vi "DAS_DEVEL.vi"() -> ()   [LabVIEW 2012]
uses:
  <vilib>/Utility/error.llb/DialogType.ctl
  SITK/Documents/SIToolkit/LabVIEW/Examples2012_4_1_0_4/Open-Close/CamHandle.vi
panel:
  out "Elapsed Time":u32
  in  "error in (no error) 4":errorcluster
  in  "bUseBuffer0 5":bool
  in  "bUseBuffer1 5":bool
  in  "Record 5":bool
  in  "Image Saving":u16(ring)=1 items=["Don't Save", "Save CoolSnap", "Save Pixelfly"]
  out "Slave OK?":bool
  in  "error in (no error) 3":errorcluster
  in  "bUseBuffer0 4":bool
  in  "bUseBuffer1 4":bool
  in  "Record 4":bool
  out "Entries in DB String":i32
  out "Database OK?":bool
  in  "?":bool
  in  "?":u16(ring) items=["Initialization", "Bulb Trigger (3x)", "Free Run (Both Cameras)", "Bulb Trigger (1x)"]
  in  "Image Tabs":T1(tab)
  in  "Display Image":dbl(ring) items=["2014-12-05_14;15;13"]
  out "Normalized Image":dbl[][](graph)
  out "Atoms":i16[][](graph)
  out "No Atoms":i16[][](graph)
  out "Dark Field":i16[][](graph)
  out "CoolSnap Free Run":i32[][](graph)
  out "CoolSnap Single Shot":i32[][](graph)
  in  "Image Tabs 2":T1(tab)
  out "Intensity Graph":dbl[][](graph)
  out "PF Atoms":u16[][](graph)
  out "PF No Atoms":u16[][](graph)
  out "PF Dark":u16[][](graph)
  out "PixelFly Free Run":u16[][](graph)
  out "PixelFly Single Shot":u16[][](graph)
  in  "Record 3":bool
  in  "bUseBuffer1 3":bool
  in  "bUseBuffer0 3":bool
  in  "Record 2":bool
  in  "bUseBuffer1 2":bool
  in  "bUseBuffer0 2":bool
  in  "bUseBuffer0":bool
  in  "bUseBuffer1":bool
  in  "Open StructureIn":T2={"Size"=88, "InterfaceType"=0, "Camera Number"=0, "CameraNumAtInterface"=0, "OpenFlags"=[], "OpenDWFlags"=[], "OpenPtrs"=[]}
  out "Bits/pixel":u16
  out "BufNr1":i16
  out "BufNr0":i16
  in  "error in (no error)":errorcluster
  in  "Camera Handle 2":u32
  in  "File and Display Name 2":string
  in  "error in (no error) 2":errorcluster
  in  "Errors":errorcluster
  in  "?":T3(tab)
  in  "Scaling":dbl(slide)=0.0016108638057548662 scale=0.001..0.1
  in  "PF Scale":dbl(slide)=0.9838778342396336 scale=0.001..10.0
  out "Database Output":string
  in  "ADC Gain":i32=-1 min=-1 step=1
  in  "ADC Speed":i32=-1 min=-3 step=1
  in  "Exposure (sec)":dbl format="%.3f"
  in  "Number of Images":u32=1
  in  "Number of Accumulations":u32=1
  in  "Acquire / Focus Flag":u32(ring)=2 items=["Synchronous Focus Mode"=1, "Synchronous NFrame Mode"=2, "Asynchronous Mode"=3, "Sequence Mode"=4]
  in  "Timing Mode":u32(ring)=4 items=["Free Run"=1, "Trigger First"=2, "Strobe"=3, "Bulb"=4, "Variable"=5, "Flash"=6]
  in  "Trigger Edge":u32(ring)=1 items=["Rising"=1, "Falling"=2]
  in  "Milliseconds Between Shots":u32=200
  in  "TriggerMode":u16(ring)=2 items=["Auto", "Software", "External sequence start ", "External exposure control"]
  in  "StorageMode":bool
  in  "Delay":u32=200
  in  "Exposure":u32=60
  in  "ExposureTimeBase":u16(ring)=1 items=["nanoseconds", "microseconds", "milliseconds"]
  in  "DelayTimeBase":u16(ring)=2 items=["nanoseconds", "microseconds", "milliseconds"]
  in  "ROIX0":u16=1 min=1
  in  "ROIY0":u16=1 min=1
  in  "ROIY1":u16=1 min=1
  in  "ROIX1":u16=1 min=1
  in  "Rate":i32
  in  "InterfaceType":u16(ring)=6 items=["IEEE1394 - Firewire", "IEEE1394/Firewire", "Matrox Helios Camera Link", "Silicon Software ME3 Camera Link", "National Instruments Camera Link", "Gigabit Ethernet", "USB", "Reserved", "Reserved", "Reserved", "Generic Camera Link with CLSER.DLL"]
  out "Top of Chamber Monitor":dynamicdata(graph)
  out "Bottom Cage Intensity Monitor":dynamicdata(graph)
  # "Stop Button"
  # "DAS Mode Select"
  # "Always run once in initialization mode before\nswitching modes. Be sure to change the camera\nsettings before running in a new mode."
  # "Images can only be saved when running \nin Bulb Trigger (3x) mode."
  # "CoolSnap HQ"
  # "CoolSnap HQ"
  # "CoolSnap HQ"
  # "CoolSnap HQ"
  # "CoolSnap HQ"
  # "CoolSnap HQ"
  # "PixelFly"
  # "PixelFly"
  # "PixelFly"
  # "PixelFly"
  # "PixelFly"
  # "PixelFly"
  # "Basic Setup"
  # "For Free Run:\n1) Synchronous Focus Mode\n2) Timing Mode: Free Run\n\nFor Bulb Trigger:\n1) Synchronous NFrame Mode\n2) Timing Mode: Bulb Trigger"
  # "Triggering Setup"
  # "Advanced Setup"
  # "For everyday use, Number of Accumulations should be 1"
  # "Basic Setup for PixelFly"
  # "For Free Run:\n1) Trigger Mode: Auto\n\nFor Bulb Trigger:\n1) Trigger Mode: External Sequence Start"
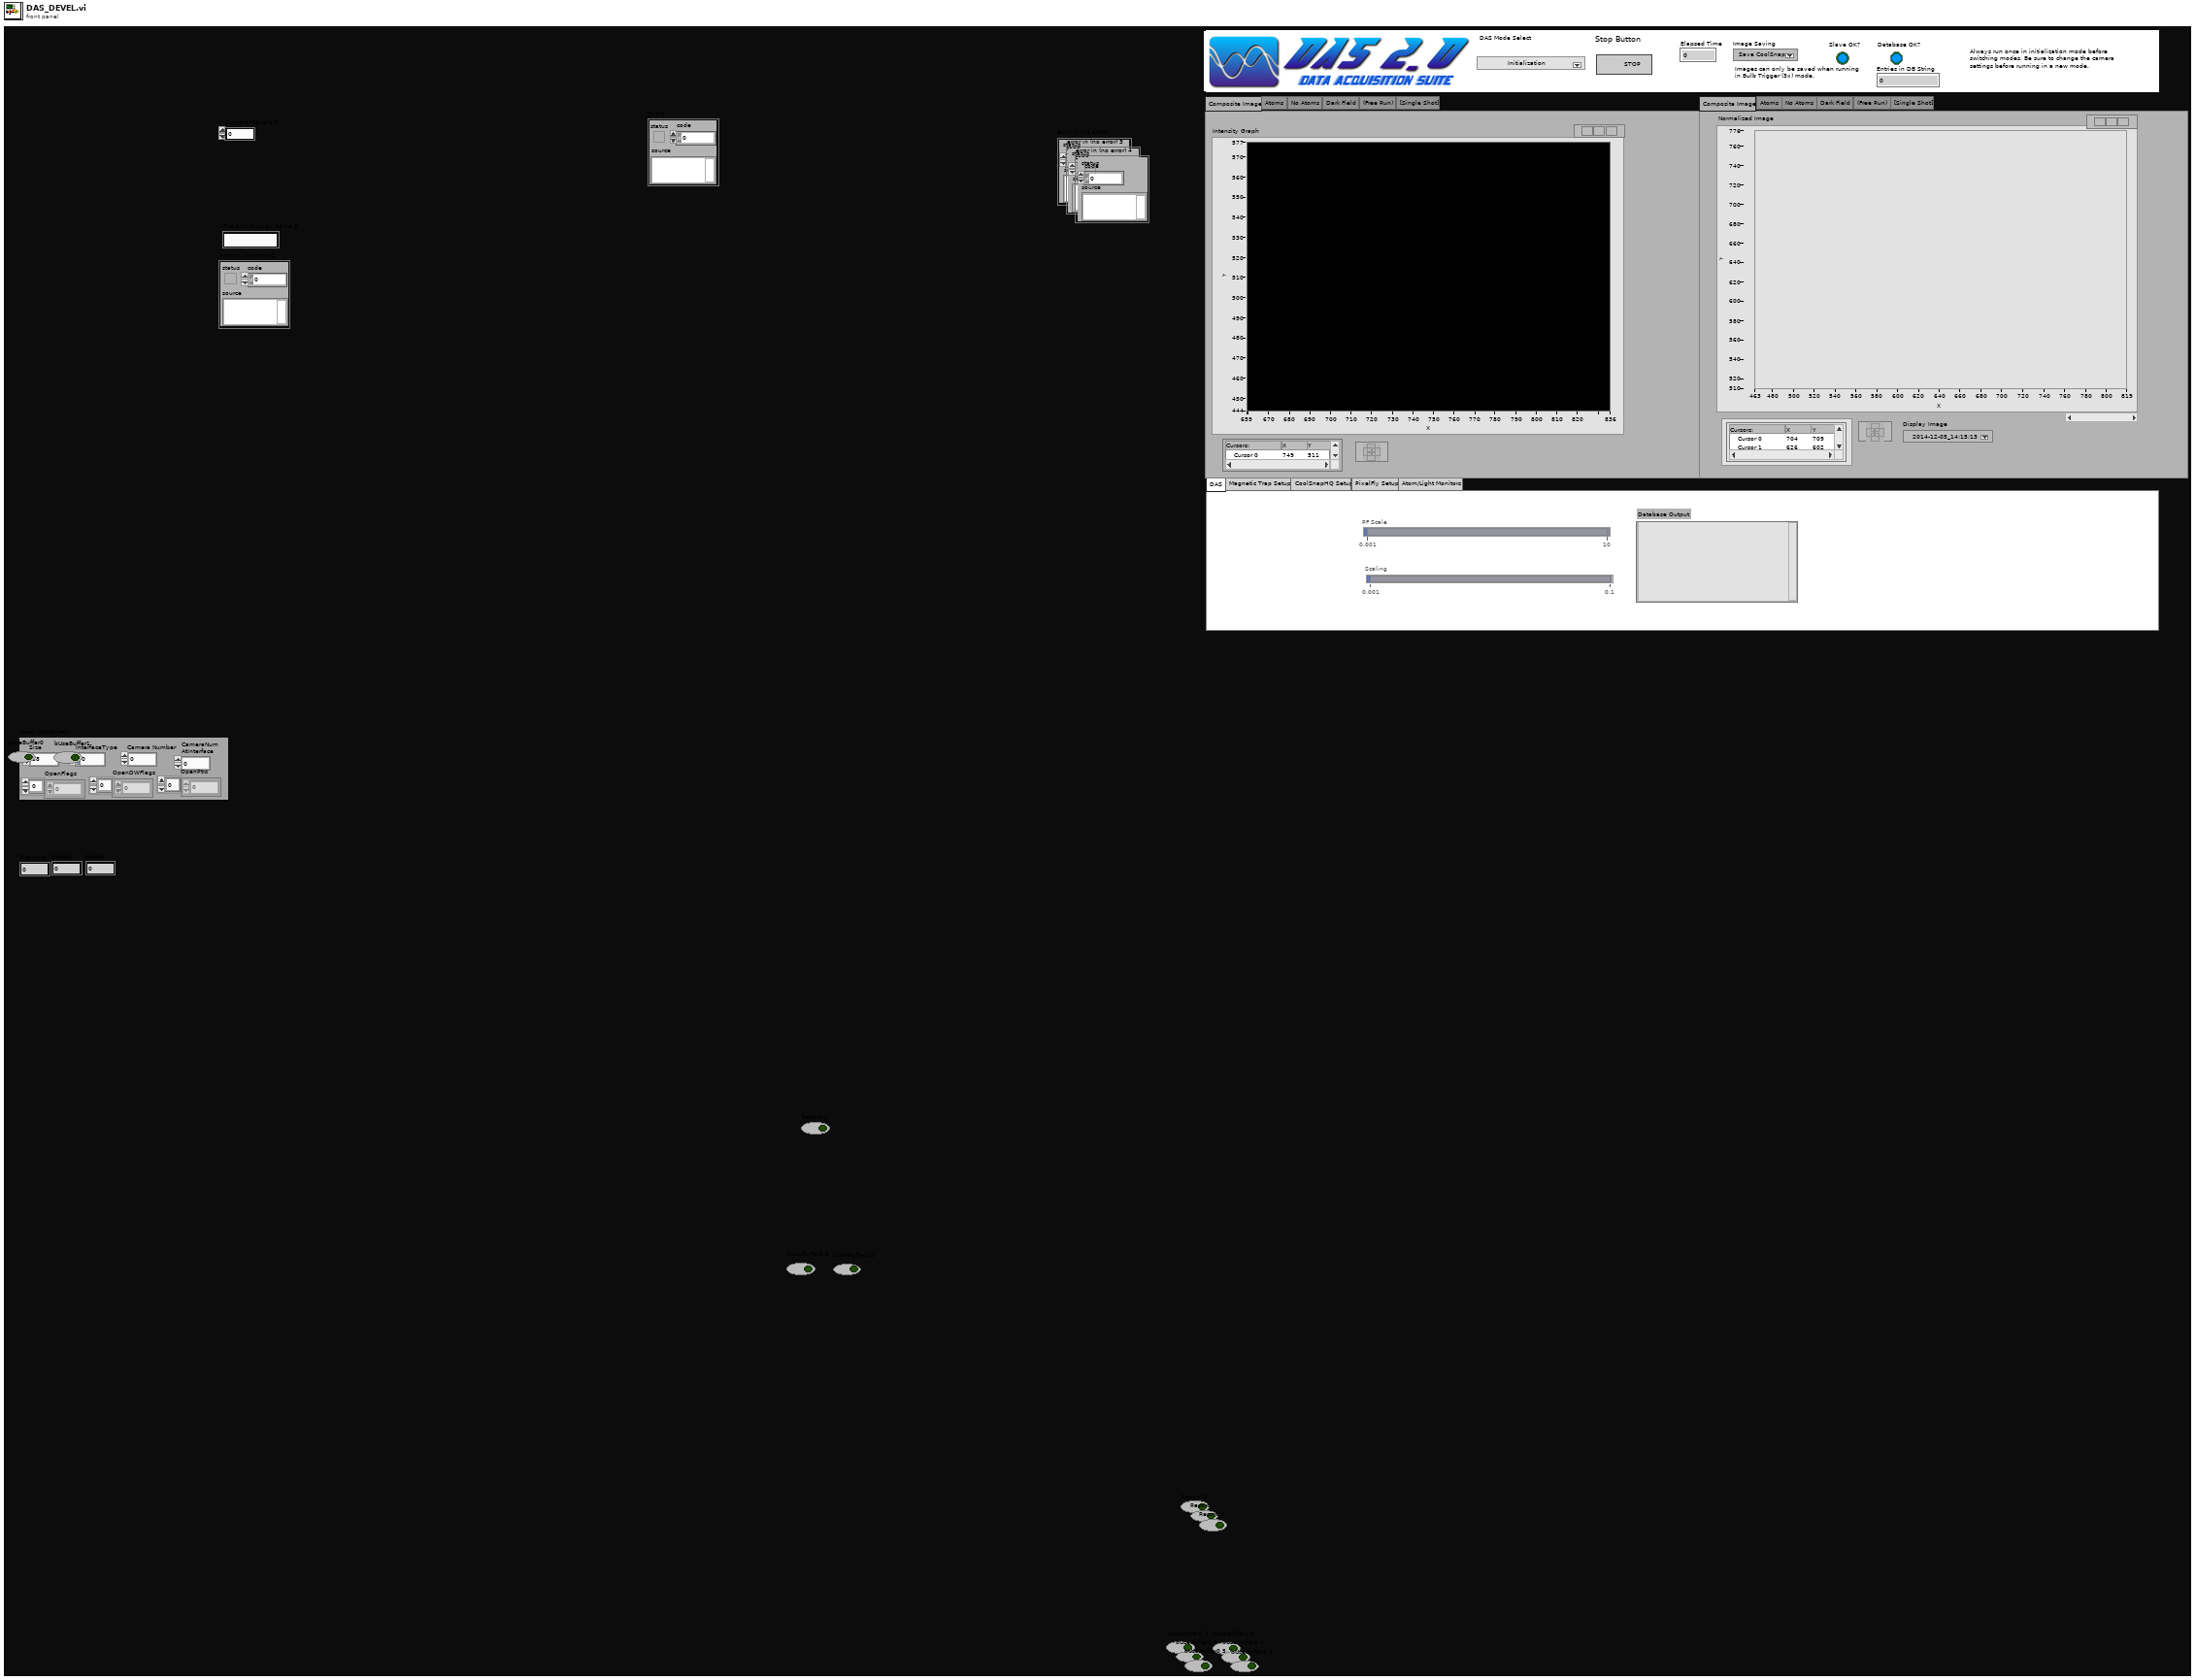
[diagram p1: front panel]
types:
  T1 = enum32{"Composite Image", "Atoms", "No Atoms", "Dark Field", "(Free Run)", "[Single Shot]"}
  T2 = cluster{"Size":u16, "InterfaceType":u16, "Camera Number":u16, "CameraNumAtInterface":u16, "OpenFlags":u16[], "OpenDWFlags":u32[], "OpenPtrs":u32[]}
  T3 = enum32{"DAS", "Magnetic Trap Setup", "CoolSnapHQ Setup", "PixelFly Setup", "Atom/Light Monitors"}
  T4 = enum16{"open", "replace", "create", "open or create", "replace or create", "replace or create with confirmation"}
  T5 = enum16{"big-endian, network order", "native, host order", "little-endian"}
  T6 = typedef "DialogType.ctl" = u16
  T7 = cluster{"Size":u16, "CamType":u16, "CamSubType":u16, "SerialNumber":u32, "HWVersion":u32, "FWVersion":u32, "InterfaceType":u16, "HardwareVersion":cluster{"BoardNum":u16, "HWVersions":cluster{"BoardName":string, "BatchNumber":u16, "MinorRevision":u8, "MajorRevision":u8, "Variant":u16}[]}, "FirmwareVersion":cluster{"DeviceNum":u16, "FWVersions":cluster{"DeviceName":string, "MinorRevision":u8, "MajorRevision":u8, "Variant":u16}[]}}
  T8 = cluster{"Size":u16, "SensorTypeDESC":u16, "SensorSubtypeDESC":u16, "MaxHorizontalResStdDESC":u16, "MaxVerticalResStdDESC":u16, "MaxHorizontalResExtDESC":u16, "MaxVerticalResExtDESC":u16, "DynResDESC":u16, "MaxBinHorzDESC":u16, "BinHorzStepDESC":bool, "MaxBinVertDESC":u16, "BinVertStepDESC":bool, "ROIHorzStepDESC":u16, "ROIVertStepDESC":u16, "NumADCDESC":u16, "IRDESC":bool, "MinDelayDESC":u32, "MaxDelayDESC":u32, "MinDelayStepDESC":u32, "MinExpoDESC":u32, "MaxExpoDESC":u32, "MinExpoStepDESC":u32, "MinDelayIRDESC":u32, "MaxDelayIRDESC":u32, "MinExpoIRDESC":u32, "MaxExpoIRDESC":u32, "TimeTableDESC":bool, "DoubleImageDESC":bool, "MinCoolSetDESC":i16, "MaxCoolSetDESC":i16, "MDefaultCoolSetDESC":i16, "PowerDownModeDESC":bool, "OffsetRegDESC":bool, "ColorPattern":cluster{"UpperLeftColor":u8, "UpperRightColor":u8, "LowerLeftColor":u8, "LowerRightColor":u8}, "PatternTypeDESC":bool, "PixelRates":u32[], "CoversionFactors":u16[], "Reserved":u32[], "NoiseFilterCapable":bool, "HotPixelCapable":bool, "HotPixelWithNoiseFilter":bool, "ASCIITimeCapable":bool, "Extended Description":bool, "Get Extended":bool, "Reserved Flag 1":bool, "Reserved Flag 2":bool}
  T9 = cluster{"Camera Handle":u32, "File Handle":u32, "Display Handle":u32, "Image Handle":u32}
  T10 = cluster{u16[][], "XResAct":u16, "YResAct":u16, "BufNrOut":i16, "BufNrOut":i16, "ErrorOut":errorcluster, "hout":u64, "Bits/pixel":u16}
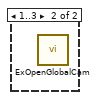
[diagram p3: hidden frame]
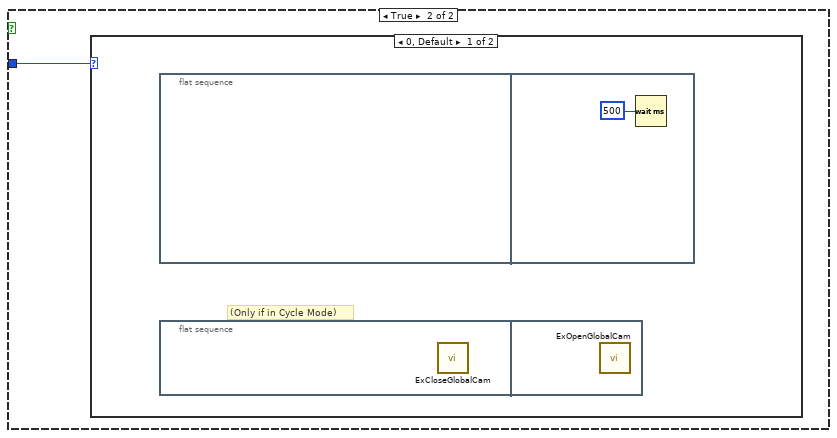
[diagram p4: hidden frame]
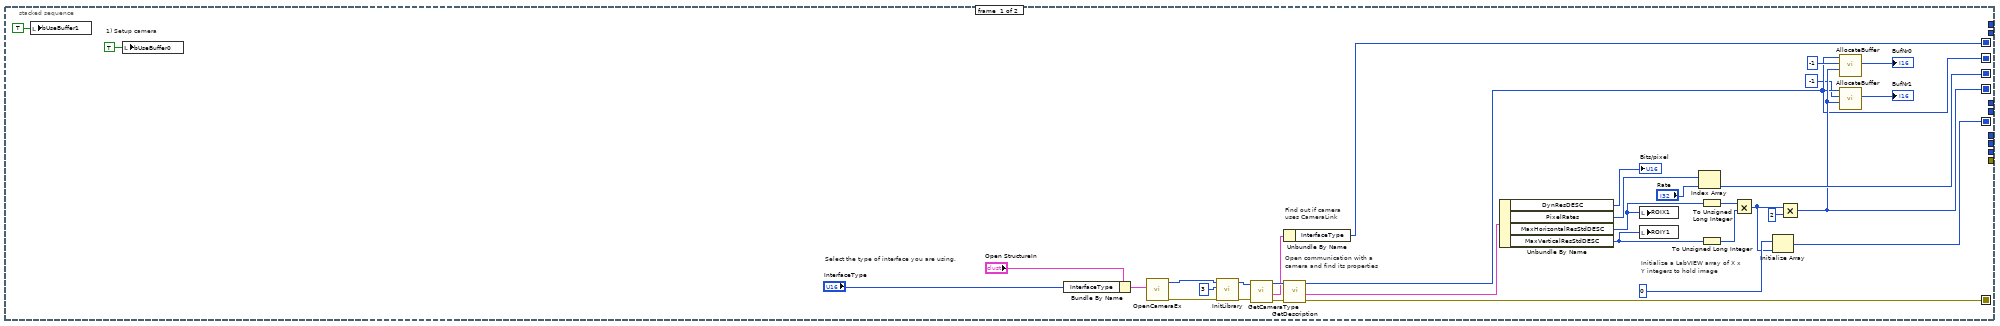
[diagram p6: hidden frame]
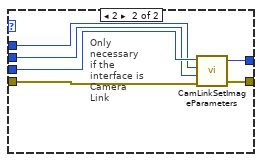
[diagram p7: hidden frame]
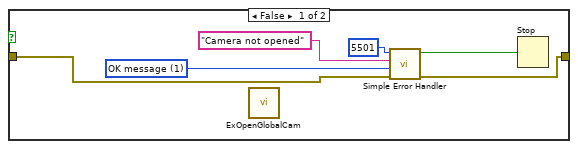
[diagram p9: hidden frame]
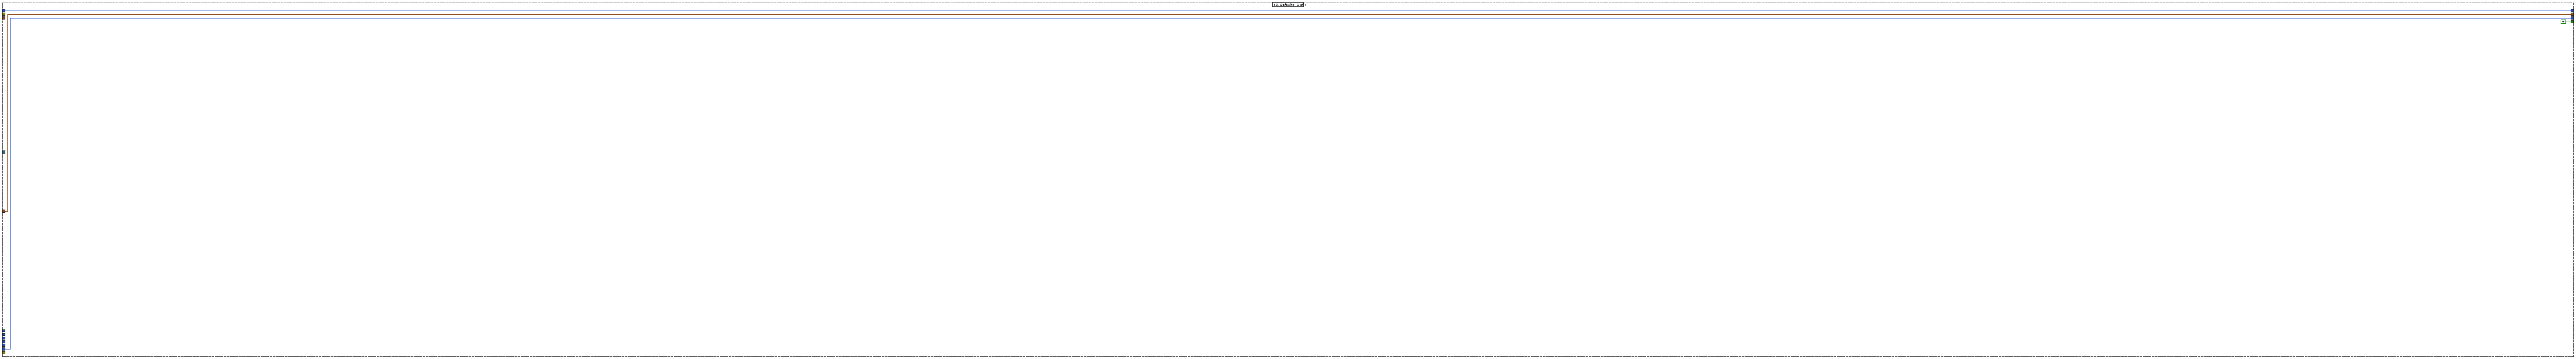
[diagram p10: hidden frame]
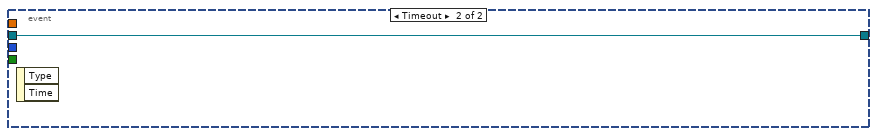
[diagram p13: hidden frame]
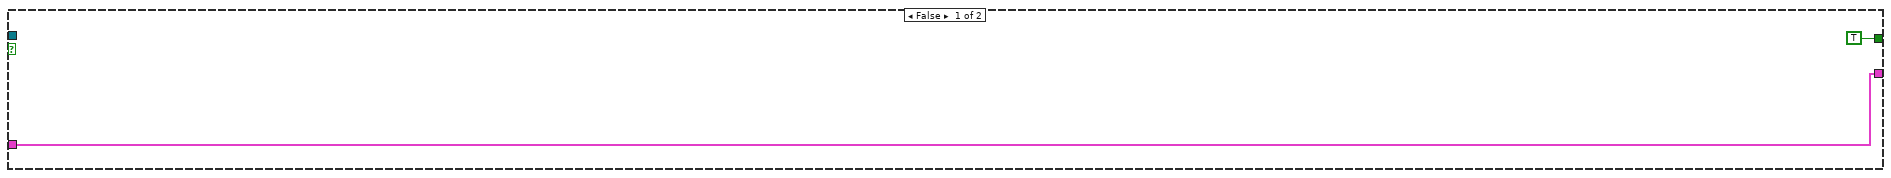
[diagram p14: hidden frame]
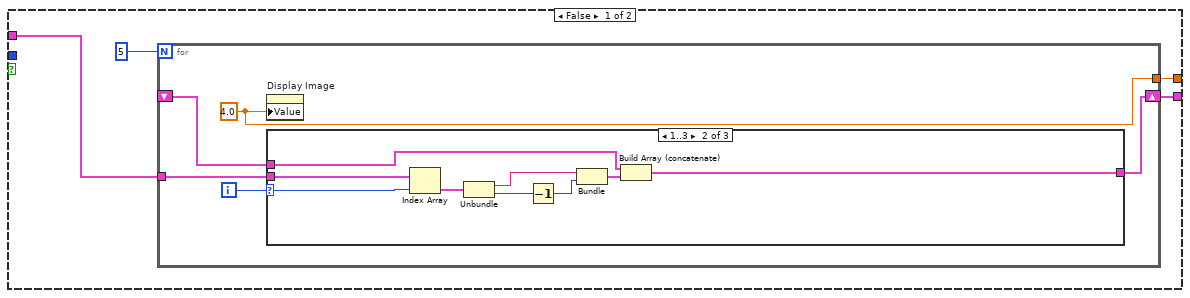
[diagram p16: hidden frame]
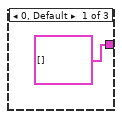
[diagram p17: hidden frame]
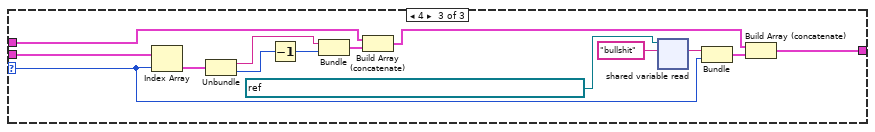
[diagram p18: hidden frame]
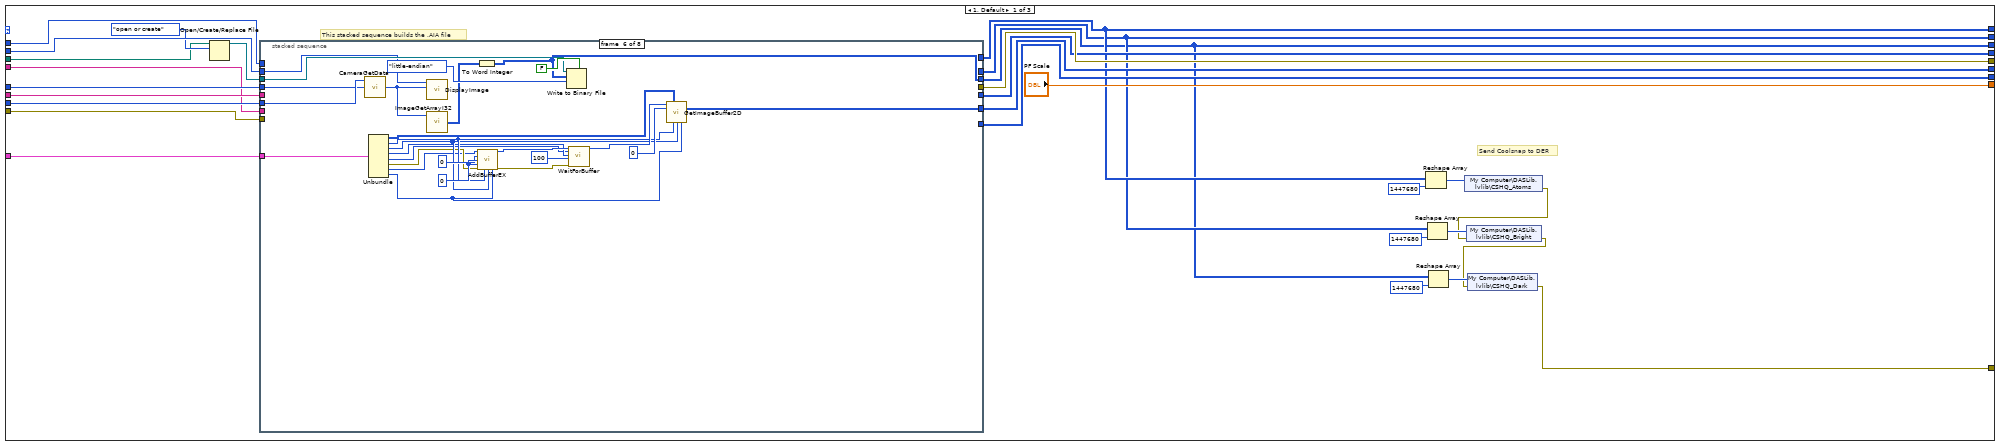
[diagram p20: hidden frame]
diagram:
  # "Tabs (Don't Touch These)"
  n1 = stacked-sequence {
    tunnel: [TRUE _] -> _
    tunnel: "?" -> [w3 _]
    tunnel: "?" -> [_ w51]
    frame #0 {
      # "Also, close any open displays to clean up the screen."
      # "Step 1:\nOpen the camera's global handle, if it is not already open."
      n2 = for {
        N: 10 -> [_]
        i -> [w8]
        w6 = T6 0 items=["no dialog", "OK message", "continue or stop message", "OK message + warnings", "continue/stop + warnings"] ("type of dialog (OK msg:1)")
        n3 = call <userlib>:"DisplayClose.vi"("Display Handle"=w8) -> ("error out"=w7:errorcluster)  [unwired: 1 in]
        n4 = call <vilib>:"General Error Handler.vi"("type of dialog (OK msg:1)"=w6, "error in (no error)"=w7) -> ()  [unwired: 9 in, 5 out]
      }
      n5 = global read "CamHandle.vi" "Camera Opened"() -> (w2:bool)
      n6 = case shown="False" w2 {
        tunnel: w3 -> [w9 w11]
        frame False {
          n7 = case shown="0, Default" w9 {
            frame 0, Default {
              n8 = flat-sequence {
                frame #0 {
                }
                frame #1 {
                  n9 = call <vilib>:"System Exec.vi"("command line"="\"C:\\Program Files\\Photometrics\\PVCam32\\utilities\\RSConfig\\RSConfig.exe\"") -> ()  [unwired: 7 in, 4 out]
                }
                frame #2 {
                  n10 = call "ExOpenGlobalCam.vi"() -> ()  [unwired: 1 in]
                }
              }
            }
            frame 1..3 {
              n11 = call "ExOpenGlobalCam.vi"() -> ()  [unwired: 1 in]
            }
          }
        }
        frame True {
          n12 = case shown="0, Default" w11 {
            frame 0, Default {
              # "(Only if in Cycle Mode)"
              n13 = flat-sequence {
                frame #0 {
                }
                frame #1 {
                  n14 = Wait (ms)(milliseconds to wait=u32 500) -> ()  [unwired: 1 out]
                }
              }
              n15 = flat-sequence {
                frame #0 {
                  n16 = call "ExCloseGlobalCam.vi"() -> ()  [unwired: 1 in]
                }
                frame #1 {
                  n17 = call "ExOpenGlobalCam.vi"() -> ()  [unwired: 1 in]
                }
              }
            }
            frame 1..3 {
            }
          }
        }
      }
    }
    frame #1 {
      w26 = u32 1  # Number Of Frames
      w27 = u32 4  # Display Type
      w28 = u32 2  # Data Type
      w30 = 13  # File Operations
      w31 = 67371008  # File Type
      w66 = u16 0 items=["Stop", "Run"] ("RecordingState")
      # "Create the Vision and Motion toolkit image(s)"
      # "Init the queue flags to FALSE"
      # "Initialize the CoolSnap Queues"
      # "Init for CoolSnap"
      # "Error Checking Sequence for CoolSnap\nCamera:"
      # "Initialization Sequence \nFor CoolSnap Camera:"
      # "This file not used"
      # "\"Build\" image and display handles"
      # "Set up display"
      # "Set up display"
      # "Step 2:\nSet up the experiment and take the images."
      # "For best performance."
      # "Execution:\n1) Outer case structure depends on DAS's state. When 0 (initialization), there is no DAQ loop.\n2) Main while loop is where DAQ and camera polling occur.\n3) Inner case structure responds to available images on camera. Hard-coded to build 3-image composite .AIA files.\n4) Innermost stacked sequence builds this .AIA file."
      # "CoolSnapHQ"
      # "Stop recording"
      n18 = flat-sequence {
        tunnel: ["Number of Images"] -> w59
        tunnel: [w183] -> w58
        tunnel: [w182] -> w57
        tunnel: [w197] -> w55
        tunnel: [w201] -> _
        tunnel: w59 -> [w201]
        tunnel: w58 -> [w200]
        tunnel: w57 -> [w199]
        tunnel: [w198] -> w54
        frame #0 {
        }
        frame #1 {
          n19 = global read "CamHandle.vi" "Cam Handle"() -> (w177:u32)
          n20 = call <userlib>:"CameraStop.vi"("Camera Handle"=w177) -> ("Camera Handle"=w178:u32)  [unwired: 1 in, 1 out]
          n21 = call <userlib>:"CameraADCset.vi"("ADC Gain"="ADC Gain", "ADC Speed"="ADC Speed", "Camera Handle"=w178) -> ("error out"=w194:errorcluster, "Camera Handle"=w196:u32)  [unwired: 3 in]
          n22 = call <userlib>:"CameraExperiment.vi"("Number of Accumulations"="Number of Accumulations", "Acquire / Focus Flag"="Acquire / Focus Flag", "error in"=w194, "Number of Images"="Number of Images", "Exposure (sec)"="Exposure (sec)", "Camera Handle"=w196) -> ("error out"=w188:errorcluster, "Camera Handle"=w189:u32)
          n23 = call <userlib>:"CameraTrigger.vi"("error in"=w188, "Trigger Edge"="Trigger Edge", "Timing Mode"="Timing Mode", "Camera Handle"=w189) -> ("error out"=w179:errorcluster, "Camera Handle"=w184:u32)
          n24 = call <userlib>:"CameraInitialize.vi"("error in"=w179, "Camera Handle"=w184) -> ("error out"=w181:errorcluster, "Camera Handle"=w180:u32)
          n25 = call <userlib>:"CameraStart.vi"("error in"=w181, "Camera Handle"=w180) -> ("error out"=w182:errorcluster, "Camera Handle"=w183:u32)
        }
        frame #2 {
          n26 = call <userlib>:"CameraCheckData.vi"("Camera Handle"=w200, "error in"=w199) -> ("Camera Handle"=w197:u32, "error out"=w198:errorcluster)  [unwired: 1 out]
        }
      }
      n27 = stacked-sequence {
        seq-local: [w100 _] -> [_ w158]
        seq-local: [w81 _] -> [_ _]
        seq-local: [w93 _] -> [_ w160]
        seq-local: [w80 _] -> [_ w155]
        seq-local: [w92 _] -> [_ w161]
        seq-local: [w91 _] -> [_ w159]
        tunnel: [_ w154] -> w50
        tunnel: [_ w150] -> w49
        tunnel: [_ w153] -> w48
        tunnel: [_ w152] -> w47
        tunnel: [_ w151] -> w46
        tunnel: [_ w149] -> w45
        tunnel: [_ w148] -> w44
        tunnel: [_ w147] -> w43
        frame #0 {
          # "Select the type of interface you are using."
          # "1) Setup camera"
          # "Find out if camera uses CameraLink"
          # "Initialize a LabVIEW array of X x Y integers to hold image"
          # "Open communication with a camera and find its properties"
          n28 = local write "bUseBuffer1"(TRUE) -> ()
          n29 = local write "bUseBuffer0"(TRUE) -> ()
          n30 = Bundle By Name(cluster="Open StructureIn", "InterfaceType"="InterfaceType") -> (w88:T2)
          n31 = call "OpenCameraEx.vi"("OpenStructureIn"=w88) -> ("error out"=w72:errorcluster, "hout"=w73:u64)  [unwired: 3 in, 2 out]
          n32 = call "InitLibrary.vi"("error in (no error)"=w72, "InterfaceType"=u32 3, "ph"=w73) -> ("error out"=w70:errorcluster, "hout"=w71:u64)  [unwired: 7 in]
          n33 = call "GetCameraType.vi"("ph"=w71, "error in (no error)"=w70) -> ("hout"=w97:u64, "CameraType"=w95:T7, "error out"=w96:errorcluster)  [unwired: 1 in, 1 out]
          n34 = Unbundle By Name(w95) -> ("InterfaceType"=w91:u16)
          n35 = call "GetDescription.vi"("ErrorIn"=w96, "ph"=w97) -> ("ErrorOut"=w92:errorcluster, "Description"=w99:T8, "hout"=w80:u64)  [unwired: 2 in, 1 out]
          n36 = Unbundle By Name(w99) -> ("DynResDESC"=→"Bits/pixel":u16, "PixelRates"=w94:u32[], "MaxHorizontalResStdDESC"=w86:u16, "MaxVerticalResStdDESC"=w85:u16)
          n37 = local write "ROIX1"(w86) -> ()
          n38 = local write "ROIY1"(w85) -> ()
          n39 = Index Array(array=w94, index="Rate") -> (element=w93:u32)
          n40 = To Unsigned Long Integer(number=w86) -> (unsigned 32bit integer=w83:u32)
          n41 = To Unsigned Long Integer(number=w85) -> (unsigned 32bit integer=w82:u32)
          n42 = Multiply(x=w83, y=w82) -> (x*y=w101:u32)
          n43 = Initialize Array(u16 0 ("Element Data"), w101) -> (w100:u16[])
          n44 = Multiply(x=w101, y=u32 2) -> (x*y=w81:u32)
          n45 = call "AllocateBuffer.vi"("Size"=w81, "BufNr"=i16 -1, "ph"=w80) -> ("BufNrOut"=→"BufNr0":i16)  [unwired: 3 in, 5 out]
          n46 = call "AllocateBuffer.vi"("Size"=w81, "BufNr"=-1, "ph"=w80) -> ("BufNrOut"=→"BufNr1":i16)  [unwired: 3 in, 5 out]
        }
        frame #1 {
          w146 = u16 1 items=["Stop", "Run"] ("RecordingState")
          # "Init for Pixelfly"
          # "Record images"
          # "Start recording"
          # "Allocate a buffer to store image data. to allocate a new buffer use buffer number = -1"
          # "Find size after arming"
          # "ArmCamera upolads all settings to the camera and prepares for new images"
          # "Find out if camera is recording, and stop it if it is"
          # "If required, insert more functions for binning.  etc. here"
          # "X x Y x 2 = number of bytes to store 1 image"
          # "Use a buffer queue to view images while recording. This is also used as \"live\" mode"
          # "Display while recording:"
          n47 = call "SetPixelRate.vi"("error in (no error)"=w161, "PixelRate"=w160, "ph"=w155) -> ("error out"=w144:errorcluster, "hout"=w145:u64)  [unwired: 2 in, 1 out]
          n48 = call "SetStorageMode.vi"("error in (no error)"=w144, "StorageMode"="StorageMode", "ph"=w145) -> ("error out"=w136:errorcluster, "hout"=w137:u64)  [unwired: 2 in, 1 out]
          n49 = call "SetTrigger.vi"("error in (no error)"=w136, "TriggerMode"="TriggerMode", "ph"=w137) -> ("error out"=w129:errorcluster, "hout"=w130:u64)  [unwired: 2 in, 1 out]
          n50 = call "SetDelayExposureTime.vi"("ph"=w130, "Delay"="Delay", "Exposure"="Exposure", "error in (no error)"=w129, "DelayTimeBase"="DelayTimeBase", "ExposureTimeBase"="ExposureTimeBase") -> ("hout"=w118:u64, "error out"=w116:errorcluster)  [unwired: 7 in, 1 out]
          n51 = call "SetROI.vi"("ph"=w118, "ROIX0"="ROIX0", "ROIY0"="ROIY0", "ROIX1"="ROIX1", "ROIY1"="ROIY1", "error in (no error)"=w116) -> ("hout"=w117:u64, "error out"=w115:errorcluster)  [unwired: 12 in]
          n52 = call "GetRecordingState.vi"("ErrorIn"=w115, "ph"=w117) -> ("ErrorOut"=w140:errorcluster, "RecordingState"=w142:u16, "hout"=w141:u64)  [unwired: 2 in, 1 out]
          n53 = case shown="1" w142 {
            tunnel: w141 -> [w171 w175]
            tunnel: w140 -> [w170 w174]
            tunnel: [w171 w173] -> w139
            tunnel: [w170 w172] -> w138
            frame 0, Default {
            }
            frame 1 {
              w176 = u16 0 items=["Stop", "Run"] ("RecordingState")
              n54 = call "SetRecordingState.vi"("ErrorIn"=w174, "RecordingState"=w176, "ph"=w175) -> ("ErrorOut"=w172:errorcluster, "hout"=w173:u64)  [unwired: 2 in, 1 out]
            }
          }
          n55 = local write "bUseBuffer0"(TRUE) -> ()
          n56 = local write "bUseBuffer1"(TRUE) -> ()
          n57 = call "ArmCamera.vi"("error in (no error)"=w138, "ph"=w139) -> ("error out"=w134:errorcluster, "hout"=w135:u64)  [unwired: 1 in, 1 out]
          n58 = call "GetSizes.vi"("ph"=w135, "ErrorIn"=w134) -> ("hout"=w131:u64, "XResAct"=w150:u16, "YResAct"=w153:u16, "ErrorOut"=w133:errorcluster)  [unwired: 11 in, 3 out]
          n59 = To Unsigned Long Integer(number=w150) -> (unsigned 32bit integer=w119:u32)
          n60 = To Unsigned Long Integer(number=w153) -> (unsigned 32bit integer=w120:u32)
          n61 = Multiply(x=w119, y=w120) -> (x*y=w121:u32)
          n62 = Multiply(x=w121, y=u32 2) -> (x*y=w106:u32)
          n63 = local read "BufNr0"() -> (w156:i16)
          n64 = call "AllocateBuffer.vi"("error in (no error)"=w133, "Size"=w106, "BufNr"=w156, "ph"=w131) -> ("error out"=w110:errorcluster, "BufNrOut"=w152:i16, "hout"=w108:u64)  [unwired: 2 in, 3 out]
          n65 = local read "BufNr1"() -> (w157:i16)
          n66 = call "AllocateBuffer.vi"("error in (no error)"=w110, "Size"=w106, "BufNr"=w157, "ph"=w108) -> ("error out"=w109:errorcluster, "BufNrOut"=w151:i16, "hout"=w107:u64)  [unwired: 2 in, 3 out]
          n67 = case shown="0, Default" w159 {
            tunnel: w109 -> [w162 w169]
            tunnel: [w162 w168] -> w124
            tunnel: w107 -> [w163 w167]
            tunnel: [w163 w166] -> w123
            tunnel: w153 -> [_ w165]
            tunnel: w150 -> [_ w164]
            frame 0, Default {
            }
            frame 2 {
              # "Only necessary if the interface is Camera Link"
              n68 = call "CamLinkSetImageParameters.vi"("error in (no error)"=w169, "YRes"=w165, "XRes"=w164, "ph"=w167) -> ("error out"=w168:errorcluster, "hout"=w166:u64)  [unwired: 1 out]
            }
          }
          n69 = local read "Bits/pixel"() -> (w147:u16)
          n70 = Reshape Array(w158, w153, w150) -> (w154:u16[][])
          n71 = call "SetRecordingState.vi"("ErrorIn"=w124, "RecordingState"=w146, "ph"=w123) -> ("ErrorOut"=w148:errorcluster, "hout"=w149:u64)  [unwired: 2 in, 1 out]
        }
      }
      n72 = Wait (ms)(milliseconds to wait=u32 5) -> ()  [unwired: 1 out]
      n73 = global read "CamHandle.vi" "Camera Opened"() -> (w41:bool)
      n74 = call <userlib>:"CameraGetDataDim.vi"("Camera Handle"="Camera Handle 2", "error in"="error in (no error) 2") -> ("Camera Handle"=w34:u32, "Xdim"=w21:u32, "Ydim"=w20:u32, "error out"=w39:errorcluster)
      n75 = while {
        tunnel: w21 -> [w210]
        tunnel: w20 -> [w209]
        tunnel: [w204] -> w25
        tunnel: [w203] -> w24
        i -> [w208]
        stop <- w205 continue-if-true
        w211 = 800
        n76 = Increment(x=w208) -> (x+1=w202:i32)
        n77 = Quotient & Remainder(x=w210, y=w202) -> (floor(x/y)=w204:u32)  [unwired: 1 out]
        n78 = Quotient & Remainder(x=w209, y=w202) -> (floor(x/y)=w203:u32)  [unwired: 1 out]
        n79 = Greater?(x=w204, y=w211) -> (0:w207:bool)
        n80 = Greater?(x=w203, y=w211) -> (0:w206:bool)
        n81 = Or(x=w207, y=w206) -> (x .or. y?=w205:bool)
      }
      n82 = case shown="True" w41 {
        tunnel: [w216 w218] -> _
        tunnel: "Errors" -> [w212 w218]
        frame False {
          w217 = u16 1 items=["no dialog", "OK message", "continue or stop message"] ("type of dialog (OK msg:1)")
          n83 = call "ExOpenGlobalCam.vi"() -> ()  [unwired: 1 in]
          n84 = call <vilib>:"Simple Error Handler.vi"("error code (no error:0)"=5501, "error source (\" \")"="Camera not opened", "type of dialog (OK msg:1)"=w217, "error in (no error)"=w212) -> ("error?"=w214:bool, "error out"=w216:errorcluster)  [unwired: 1 in, 3 out]
          n85 = Stop(stop? (T)=w214) -> ()
        }
        frame True {
        }
      }
      n86 = Obtain Queue(max queue size (-1, unlimited)=5, name (unnamed)="CSHQ_1", element data type=dbl[][] [] ("Normalized Image")) -> (queue out=w42:refnum<queue>)  [unwired: 2 in, 2 out]
      n87 = shared-variable-write(refnum<k21> "ni.var.psp://my computer/Untitled Library 1/CSHQ_1_Changed" ("shared variable refnum in"), FALSE) -> ()  [unwired: 1 in, 2 out]
      n88 = To Unsigned Long Integer(number=w25) -> (unsigned 32bit integer=w23:u32)
      n89 = To Unsigned Long Integer(number=w24) -> (unsigned 32bit integer=w22:u32)
      n90 = call <userlib>:"ImageCreate.vi"("X dimension"=w21, "Y dimension"=w20, "Data Type"=w28, "error in"=w39, "Number Of Frames"=w26) -> ("Image Handle"=w32:u32, "error out"=w38:errorcluster)
      n91 = call <userlib>:"DisplayOpen.vi"("Display Title"="File and Display Name 2", "Image Handle"=w32, "error in"=w38, "Display Height"=w22, "Display Width"=w23, "Display Type"=w27) -> ("error out"=w37:errorcluster, "Display Handle"=w18:u32)
      n92 = call <userlib>:"FileOpen.vi"("error in"=w37, "File Operations"=w30, "FileName"="File and Display Name 2", "File Type"=w31) -> ("File Handle"=w33:u32)  [unwired: 1 out]
      n93 = Bundle("Camera Handle"=w34, "File Handle"=w33, "Display Handle"=w18, "Image Handle"=w32) -> (w53:T9)  [unwired: 1 in]
      n94 = Bundle("Xdim"=w21, "Ydim"=w20, 0) -> (w56:cluster{"Xdim":u32, "Ydim":u32, i32})  [unwired: 1 in]
      n95 = case shown="1" w51 {
        selector: w51 -> [_ w234 w1045 w1132]
        tunnel: w53 -> [w222 w236 w1047 w1134]
        tunnel: [w222 w236 w1047 w1134] -> w69
        tunnel: w55 -> [w221 w241 w1052 w1139]
        tunnel: w54 -> [_ _ _ _]
        tunnel: [w221 w241 w1052 w1139] -> _
        tunnel: [TRUE FALSE FALSE FALSE] -> _
        tunnel: w56 -> [_ _ _ _]
        tunnel: w50 -> [_ w233 w1044 w1131]
        tunnel: w49 -> [_ w232 w1043 w1130]
        tunnel: w48 -> [_ w231 w1042 w1129]
        tunnel: w47 -> [_ w230 w1041 w1128]
        tunnel: w46 -> [_ w229 w1040 w1127]
        tunnel: w45 -> [w219 w228 w1039 w1126]
        tunnel: w44 -> [_ w227 w1038 w1125]
        tunnel: w43 -> [_ w226 w1037 w1124]
        tunnel: [w219 w225 w1036 w1123] -> w65
        tunnel: w42 -> [_ w224 _ _]
        frame 0, Default {
        }
        frame 1 {
          n96 = Unbundle(w236) -> ("Camera Handle"=w235:u32, "File Handle"=w239:u32, "Display Handle"=w238:u32, "Image Handle"=w237:u32)
          n97 = while {
            tunnel: "error in (no error)" -> [w290]
            tunnel: w235 -> [w289]
            tunnel: [w286] -> _
            tunnel: w239 -> [_]
            tunnel: w238 -> [w285]
            tunnel: w237 -> [w284]
            tunnel: [w282] -> _
            tunnel: w234 -> [w276]
            tunnel: w233 -> [w272]
            tunnel: w232 -> [w271]
            tunnel: w231 -> [w270]
            tunnel: w230 -> [w268]
            tunnel: w229 -> [w269]
            tunnel: w228 -> [w264]
            tunnel: w227 -> [w267]
            tunnel: w226 -> [w266]
            tunnel: [w264] -> w225
            shift-right: [w263] -> _
            shift-left: w224 -> [w249]
            shift-right: [w256] -> _
            shift-left: cluster{"date/time string":string, i32}[] [] -> [w257]
            stop <- w275 continue-if-true
            (unwired) 1
            # "Destroy the buffer,\nfind the right image,\nrebuild the buffer"
            # "Cluster for PixelFly"
            # "PixelFly Camera Functions"
            # "NI Scope"
            # "CoolSnap Camera Functions"
            # "ADC Inputs"
            # "THIS is the main loop.\nPoll the camera continuously while other data is taken in."
            n98 = Bundle(w272, "XResAct"=w271, "YResAct"=w270, "BufNrOut"=w269, "BufNrOut"=w268, "ErrorOut"=w267, "hout"=w264, "Bits/pixel"=w266) -> (w265:T10)  [unwired: 1 in]
            n99 = call <userlib>:"CameraCheckData.vi"("Camera Handle"=w289, "error in"=w290) -> ("Camera Handle"=w288:u32, "Number Of Frames Available"=w281:i32, "error out"=w287:errorcluster)
            n100 = Wait Until Next ms Multiple(millisecond multiple=1) -> (millisecond timer value=w282:u32)
            "Elapsed Time" <- w282
            n101 = Not(x="?") -> (.not. x?=w274:bool)
            n102 = Greater Or Equal?(x=w281, y=1) -> (x >= y?=w279:bool)
            n103 = Greater?(x=w276, y=u16 0) -> (0:w247:bool)
            n104 = call "DAQ Assistant"() -> ("data"=w243:dynamicdata)  [unwired: 17 in, 2 out]
            n105 = And(x=w247, y=w274) -> (x .and. y?=w275:bool)
            n106 = Split Signals(w243) -> (w245:dynamicdata, →"Bottom Cage Intensity Monitor":dynamicdata)  [unwired: 2 in]
            n107 = case shown="True" w279 {
              selector: w279 -> [w387 _]
              tunnel: w288 -> [_ w456]
              tunnel: w287 -> [w388 w455]
              tunnel: [w387 TRUE] -> _
              tunnel: [w388 w448] -> w286
              tunnel: w285 -> [_ w454]
              tunnel: w284 -> [_ w451]
              tunnel: w282 -> [_ _]
              tunnel: w265 -> [_ w440]
              tunnel: w249 -> [w386 w418]
              tunnel: [w386 w416] -> w250
              tunnel: "Image Saving" -> [_ w411]
              frame False {
              }
              frame True {
                w422 = 0 ("y")
                # "Enter this loop when image data is available on the coolsnap"
                # "Add new image to \"top\" of queue"
                # "Save Images?"
                n108 = Get Queue Status(queue=w418) -> (queue out=w417:refnum<queue>, # elements in queue=w421:i32)  [unwired: 2 in, 6 out]
                n109 = Less?(x=w421, y=5) -> (x < y?=w419:bool)
                n110 = Get Date/Time In Seconds() -> (seconds since 1Jan1904=w442:timestamp)
                n111 = Format Date/Time String(time format string (%c)="%Y-%m-%d_%H;%M;%S", seconds (now)=w442) -> (date/time string=w413:string)  [unwired: 1 in]
                n112 = Concatenate Strings("Z:\\Current\\" ("string"), w413, ".aia" ("string")) -> (w449:string)
                n113 = String To Path(string=w449) -> (path=w410:path)
                n114 = call <vilib>:"System Exec.vi"("command line"="php C:\\Users\\BECV\\Documents\\GitHub\\DAS\\dbquery.php") -> ("standard output"=w399:string)  [unwired: 7 in, 3 out]
                n115 = case shown="2" w411 {
                  tunnel: w456 -> [w484 w669 w851]
                  tunnel: w455 -> [w483 w668 w850]
                  tunnel: w454 -> [w482 w667 w849]
                  tunnel: w451 -> [w481 w666 w848]
                  tunnel: w410 -> [w471 w657 _]
                  tunnel: [w480 w665 w841] -> w448
                  tunnel: "Milliseconds Between Shots" -> [w479 w664 w847]
                  tunnel: w440 -> [w478 w663 w846]
                  tunnel: [w459 w662 w830] -> w395
                  tunnel: [w458 w661 w829] -> w394
                  tunnel: [w457 w660 w827] -> w392
                  tunnel: [w477 w644 w845] -> w435
                  tunnel: [w476 w643 w844] -> w432
                  tunnel: [w475 w642 w828] -> w429
                  tunnel: ["PF Scale" w654 w840] -> w426
                  tunnel: w413 -> [w469 w655 w843]
                  tunnel: w399 -> [w473 w659 w842]
                  tunnel: [w460 w645 errorcluster {"status"=FALSE, "code"=0, "source"=""} ("error IO")] -> w391
                  frame 1, Default {
                    # "Send Coolsnap to DER"
                    # "This stacked sequence builds the .AIA file"
                    n116 = Open/Create/Replace File(file path (use dialog)=w471, operation (0:open)=T4."open or create") -> (refnum out=w470:refnum<file>)  [unwired: 4 in, 2 out]
                    n117 = stacked-sequence {
                      tunnel: w484 -> [_ w538 _ w571 _ w601 _ _]
                      tunnel: w483 -> [_ _ _ _ _ _ _ _]
                      tunnel: w482 -> [_ w540 _ w568 _ w598 _ _]
                      tunnel: w481 -> [_ w539 _ w567 _ w597 _ _]
                      tunnel: w470 -> [w498 w532 _ w569 _ w599 w610 w641]
                      tunnel: [_ w535 _ _ _ _ _ _] -> w480
                      tunnel: w479 -> [_ _ w542 _ w572 _ _ _]
                      tunnel: [_ w516 _ _ _ _ _ _] -> w459
                      tunnel: [_ _ _ w563 _ _ _ _] -> w458
                      tunnel: [_ _ _ _ _ w593 _ _] -> w457
                      tunnel: w478 -> [_ w500 _ w547 _ w577 _ _]
                      tunnel: [_ w499 _ _ _ _ _ _] -> w477
                      tunnel: [_ _ _ w546 _ _ _ _] -> w476
                      tunnel: [_ _ _ _ _ w576 _ _] -> w475
                      tunnel: w469 -> [_ _ _ _ _ _ w608 _]
                      tunnel: w473 -> [_ _ _ _ _ _ w604 _]
                      frame #0 {
                        # "AIA, 16 bit, NULL"
                        n118 = Write to Binary File(file (use dialog)=w498, data="AIA", 5:FALSE ("prepend array or string size? (T)"), 9:T5."little-endian" ("byte order (0:big-endian, network order)")) -> (refnum out=w494:refnum<file>)  [unwired: 2 in, 2 out]
                        n119 = To Byte Integer(number=2) -> (8bit integer=w487:i8)
                        n120 = Write to Binary File(file (use dialog)=w494, data=w487, 5:FALSE ("prepend array or string size? (T)"), 9:T5."little-endian" ("byte order (0:big-endian, network order)")) -> (refnum out=w493:refnum<file>)  [unwired: 2 in, 2 out]
                        n121 = To Byte Integer(number=0) -> (8bit integer=w485:i8)
                        n122 = Write to Binary File(file (use dialog)=w493, data=w485, 5:FALSE ("prepend array or string size? (T)"), 9:T5."little-endian" ("byte order (0:big-endian, network order)")) -> ()  [unwired: 2 in, 3 out]
                      }
                      frame #1 {
                        w511 = 0
                        w525 = T5."little-endian" ("byte order (0:big-endian, network order)")
                        n123 = call <userlib>:"CameraGetData.vi"("Data Handle"=w539, "Camera Handle"=w538) -> ("error out"=w541:errorcluster, "Data Handle"=w536:u32)  [unwired: 1 in, 1 out]
                        n124 = Unbundle(w500) -> (w508:u16[][], "XResAct"=w507:u16, "YResAct"=w506:u16, "BufNrOut"=w505:i16, "BufNrOut"=w504:i16, "ErrorOut"=w503:errorcluster, "hout"=w502:u64, "Bits/pixel"=w501:u16)
                        n125 = call <userlib>:"DisplayImage.vi"("error in"=w541, "Image Handle"=w536, "Display Handle"=w540) -> ()  [unwired: 1 in, 2 out]
                        n126 = call <userlib>:"ImageGetArrayI32.vi"("Image Handle"=w536) -> ("Array int 32"=w517:i32[][])  [unwired: 2 in, 2 out]
                        n127 = To Word Integer(number=w517) -> (16bit integer=w516:i16[][])
                        n128 = Array Size(array=w517) -> (size(s)=w518:i32[])
                        n129 = call "AddBufferEX.vi"("ph"=w502, "BuffNr"=i16 0, "1stImage"=w511, "LastImage"=w511, "error in (no error)"=w503, "XRes"=w507, "YRes"=w506, "BitPerPixel"=w501) -> ("hout"=w513:u64, "error out"=w512:errorcluster)  [unwired: 5 in, 1 out]
                        n130 = Index Array(array=w518, index=0) -> (element=w523:i32)
                        n131 = Index Array(array=w518, index=1) -> (element=w522:i32)
                        n132 = call "WaitForBuffer.vi"("ph"=w513, "sBufNr"=w504, "sBufNr 2"=w505, "timeout"=100, "error in (no error)"=w512) -> ("hout"=w515:u64)  [unwired: 10 in, 4 out]
                        n133 = To Word Integer(number=w523) -> (16bit integer=w524:i16)
                        n134 = To Word Integer(number=w522) -> (16bit integer=w521:i16)
                        n135 = Write to Binary File(file (use dialog)=w532, data=w524, 5:FALSE ("prepend array or string size? (T)"), 9:w525) -> (refnum out=w531:refnum<file>)  [unwired: 2 in, 2 out]
                        n136 = call "GetImageBuffer2D.vi"("ph"=w515, "BuffIn"=w508, "BuffNr"=i16 0, "xRes"=w507, "yRes"=w506, "Bitresolution"=w501) -> ("BuffOut"=w499:u16[][])  [unwired: 6 in, 3 out]
                        n137 = Write to Binary File(file (use dialog)=w531, data=w521, 5:FALSE ("prepend array or string size? (T)"), 9:w525) -> (refnum out=w530:refnum<file>)  [unwired: 2 in, 2 out]
                        n138 = To Word Integer(number=3 ("index")) -> (16bit integer=w520:i16)
                        n139 = Write to Binary File(file (use dialog)=w530, data=w520, 5:FALSE ("prepend array or string size? (T)"), 9:w525) -> (refnum out=w529:refnum<file>)  [unwired: 2 in, 2 out]
                        n140 = Write to Binary File(file (use dialog)=w529, data=w516, 5:FALSE ("prepend array or string size? (T)"), 9:w525) -> (error out=w535:errorcluster)  [unwired: 2 in, 2 out]
                      }
                      frame #2 {
                        n141 = Quotient & Remainder(x=w542, y=u32 10) -> (floor(x/y)=w543:u32)  [unwired: 1 out]
                        n142 = Add(x=w543, y=w542) -> (x+y=w545:u32)
                        n143 = Wait (ms)(milliseconds to wait=w545) -> ()  [unwired: 1 out]
                      }
                      frame #3 {
                        w558 = 0
                        n144 = call <userlib>:"CameraGetData.vi"("Data Handle"=w567, "Camera Handle"=w571) -> ("Data Handle"=w566:u32)  [unwired: 1 in, 2 out]
                        n145 = Unbundle(w547) -> (w555:u16[][], "XResAct"=w554:u16, "YResAct"=w553:u16, "BufNrOut"=w552:i16, "BufNrOut"=w551:i16, "ErrorOut"=w550:errorcluster, "hout"=w549:u64, "Bits/pixel"=w548:u16)
                        n146 = call <userlib>:"DisplayImage.vi"("Image Handle"=w566, "Display Handle"=w568) -> ()  [unwired: 2 in, 2 out]
                        n147 = call <userlib>:"ImageGetArrayI32.vi"("Image Handle"=w566) -> ("Array int 32"=w564:i32[][])  [unwired: 2 in, 2 out]
                        n148 = To Word Integer(number=w564) -> (16bit integer=w563:i16[][])
                        n149 = call "AddBufferEX.vi"("ph"=w549, "BuffNr"=i16 0, "1stImage"=w558, "LastImage"=w558, "error in (no error)"=w550, "XRes"=w554, "YRes"=w553, "BitPerPixel"=w548) -> ("hout"=w560:u64, "error out"=w559:errorcluster)  [unwired: 5 in, 1 out]
                        n150 = Write to Binary File(file (use dialog)=w569, data=w563, 5:FALSE ("prepend array or string size? (T)"), 9:T5."little-endian" ("byte order (0:big-endian, network order)")) -> ()  [unwired: 2 in, 3 out]
                        n151 = call "WaitForBuffer.vi"("ph"=w560, "sBufNr"=w551, "sBufNr 2"=w552, "timeout"=100, "error in (no error)"=w559) -> ("hout"=w562:u64)  [unwired: 10 in, 4 out]
                        n152 = call "GetImageBuffer2D.vi"("ph"=w562, "BuffIn"=w555, "BuffNr"=i16 0, "xRes"=w554, "yRes"=w553, "Bitresolution"=w548) -> ("BuffOut"=w546:u16[][])  [unwired: 6 in, 3 out]
                      }
                      frame #4 {
                        n153 = Quotient & Remainder(x=w572, y=u32 10) -> (floor(x/y)=w573:u32)  [unwired: 1 out]
                        n154 = Add(x=w573, y=w572) -> (x+y=w575:u32)
                        n155 = Wait (ms)(milliseconds to wait=w575) -> ()  [unwired: 1 out]
                      }
                      frame #5 {
                        w588 = 0
                        n156 = call <userlib>:"CameraGetData.vi"("Data Handle"=w597, "Camera Handle"=w601) -> ("Data Handle"=w596:u32)  [unwired: 1 in, 2 out]
                        n157 = Unbundle(w577) -> (w585:u16[][], "XResAct"=w584:u16, "YResAct"=w583:u16, "BufNrOut"=w582:i16, "BufNrOut"=w581:i16, "ErrorOut"=w580:errorcluster, "hout"=w579:u64, "Bits/pixel"=w578:u16)
                        n158 = call <userlib>:"DisplayImage.vi"("Image Handle"=w596, "Display Handle"=w598) -> ()  [unwired: 2 in, 2 out]
                        n159 = call <userlib>:"ImageGetArrayI32.vi"("Image Handle"=w596) -> ("Array int 32"=w594:i32[][])  [unwired: 2 in, 2 out]
                        n160 = To Word Integer(number=w594) -> (16bit integer=w593:i16[][])
                        n161 = call "AddBufferEX.vi"("ph"=w579, "BuffNr"=i16 0, "1stImage"=w588, "LastImage"=w588, "error in (no error)"=w580, "XRes"=w584, "YRes"=w583, "BitPerPixel"=w578) -> ("hout"=w590:u64, "error out"=w589:errorcluster)  [unwired: 5 in, 1 out]
                        n162 = Write to Binary File(file (use dialog)=w599, data=w593, 5:FALSE ("prepend array or string size? (T)"), 9:T5."little-endian" ("byte order (0:big-endian, network order)")) -> ()  [unwired: 2 in, 3 out]
                        n163 = call "WaitForBuffer.vi"("ph"=w590, "sBufNr"=w581, "sBufNr 2"=w582, "timeout"=100, "error in (no error)"=w589) -> ("hout"=w592:u64)  [unwired: 10 in, 4 out]
                        n164 = call "GetImageBuffer2D.vi"("ph"=w592, "BuffIn"=w585, "BuffNr"=i16 0, "xRes"=w584, "yRes"=w583, "Bitresolution"=w578) -> ("BuffOut"=w576:u16[][])  [unwired: 6 in, 3 out]
                      }
                      frame #6 {
                        # "Indicate DB\nIssue"
                        # "Number of replacements is number of lines"
                        n165 = Search and Replace String(replace all?=TRUE ("replace all? (F)"), input string=w604, search string="(") -> (result string=w614:string)  [unwired: 5 in, 3 out]
                        n166 = Search and Replace String(replace all?=TRUE ("replace all? (F)"), input string=w614, search string=")") -> (result string=w607:string, number of replacements=w602:i32)  [unwired: 5 in, 2 out]
                        "Database Output" <- w607
                        n167 = for {
                          N: w602 -> [_]
                          tunnel: w607 -> [w639]
                          tunnel: w610 -> [w635]
                          i -> [w640]
                          w627 = T5."little-endian" ("byte order (0:big-endian, network order)")
                          n168 = Pick Line(multi-line string=w639, line index=w640) -> (output string=w638:string)  [unwired: 1 in]
                          n169 = Match Pattern(string=w638, regular expression="\\s") -> (before substring=w630:string, after substring=w636:string)  [unwired: 1 in, 2 out]
                          n170 = Concatenate Strings(w630) -> (w629:string)
                          n171 = Fract/Exp String To Number(string=w636) -> (number=w624:dbl)  [unwired: 3 in, 1 out]
                          n172 = To Double Precision Float(number=w624) -> (double precision float=w622:dbl)
                          n173 = Write to Binary File(file (use dialog)=w635, data=w629, 5:FALSE ("prepend array or string size? (T)"), 9:w627) -> (refnum out=w631:refnum<file>, error out=w632:errorcluster)  [unwired: 2 in, 1 out]
                          n174 = To Byte Integer(number=0) -> (8bit integer=w621:i8)
                          n175 = Write to Binary File(file (use dialog)=w631, data=w621, error in=w632, 5:FALSE ("prepend array or string size? (T)"), 9:T5."little-endian" ("byte order (0:big-endian, network order)")) -> (refnum out=w625:refnum<file>, error out=w628:errorcluster)  [unwired: 1 in, 1 out]
                          n176 = Write to Binary File(file (use dialog)=w625, data=w622, error in=w628, 5:FALSE ("prepend array or string size? (T)"), 9:w627) -> ()  [unwired: 1 in, 3 out]
                        }
                        n177 = String Length(string=w607) -> (length=w603:i32)
                        n178 = Greater?(x=w603, y=10) -> (0:w605:bool)
                        n179 = case shown="True" w605 {
                          tunnel: w602 -> [w616 w618]
                          frame False {
                            n180 = local write "Entries in DB String"(w616) -> ()
                            n181 = local write "Database OK?"(TRUE ("Database OK?")) -> ()
                          }
                          frame True {
                            "Database OK?" <- FALSE ("Database OK?")
                            "Entries in DB String" <- w618
                          }
                        }
                        n182 = shared-variable-write(refnum<k21> "ni.var.psp://my computer/Untitled Library 1/CSHQ_1_Time" ("shared variable refnum in"), w608) -> ()  [unwired: 1 in, 2 out]
                      }
                      frame #7 {
                        n183 = Close File(refnum=w641) -> ()  [unwired: 1 in, 2 out]
                      }
                    }
                    n184 = Reshape Array(w459, 1447680 ("dimension size")) -> (w465:i16[])
                    n185 = Reshape Array(w458, 1447680 ("dimension size")) -> (w463:i16[])
                    n186 = Reshape Array(w457, 1447680 ("dimension size")) -> (w464:i16[])
                    n187 = shared-variable "My Computer\\DASLib.lvlib\\CSHQ_Atoms"(w465) -> (error out=w462:errorcluster)  [unwired: 1 in]
                    n188 = shared-variable "My Computer\\DASLib.lvlib\\CSHQ_Bright"(w463, error in=w462) -> (error out=w461:errorcluster)
                    n189 = shared-variable "My Computer\\DASLib.lvlib\\CSHQ_Dark"(w464, error in=w461) -> (error out=w460:errorcluster)
                  }
                  frame 2 {
                    # "Send Pixelfly to DER using the Coolsnap variable"
                    # "This stacked sequence builds the .AIA file"
                    n190 = Open/Create/Replace File(file path (use dialog)=w657, operation (0:open)=T4."open or create") -> (refnum out=w656:refnum<file>)  [unwired: 4 in, 2 out]
                    n191 = stacked-sequence {
                      tunnel: w669 -> [_ w723 _ w756 _ w786 _ _]
                      tunnel: w668 -> [_ _ _ _ _ _ _ _]
                      tunnel: w667 -> [_ w725 _ w753 _ w783 _ _]
                      tunnel: w666 -> [_ w724 _ w752 _ w782 _ _]
                      tunnel: w656 -> [w683 w717 _ w754 _ w784 w795 w826]
                      tunnel: [_ w720 _ _ _ _ _ _] -> w665
                      tunnel: w664 -> [_ _ w727 _ w757 _ _ _]
                      tunnel: [_ w701 _ _ _ _ _ _] -> w662
                      tunnel: [_ _ _ w748 _ _ _ _] -> w661
                      tunnel: [_ _ _ _ _ w778 _ _] -> w660
                      tunnel: w663 -> [_ w685 _ w732 _ w762 _ _]
                      tunnel: [_ w684 _ _ _ _ _ _] -> w644
                      tunnel: [_ _ _ w731 _ _ _ _] -> w643
                      tunnel: [_ _ _ _ _ w761 _ _] -> w642
                      tunnel: w655 -> [_ _ _ _ _ _ w793 _]
                      tunnel: w659 -> [_ _ _ _ _ _ w790 _]
                      frame #0 {
                        # "AIA, 16 bit, NULL"
                        n192 = Write to Binary File(file (use dialog)=w683, data="AIA", 5:FALSE ("prepend array or string size? (T)"), 9:T5."little-endian" ("byte order (0:big-endian, network order)")) -> (refnum out=w679:refnum<file>)  [unwired: 2 in, 2 out]
                        n193 = To Byte Integer(number=2) -> (8bit integer=w672:i8)
                        n194 = Write to Binary File(file (use dialog)=w679, data=w672, 5:FALSE ("prepend array or string size? (T)"), 9:T5."little-endian" ("byte order (0:big-endian, network order)")) -> (refnum out=w678:refnum<file>)  [unwired: 2 in, 2 out]
                        n195 = To Byte Integer(number=0) -> (8bit integer=w670:i8)
                        n196 = Write to Binary File(file (use dialog)=w678, data=w670, 5:FALSE ("prepend array or string size? (T)"), 9:T5."little-endian" ("byte order (0:big-endian, network order)")) -> ()  [unwired: 2 in, 3 out]
                      }
                      frame #1 {
                        w696 = 0
                        w710 = T5."little-endian" ("byte order (0:big-endian, network order)")
                        n197 = call <userlib>:"CameraGetData.vi"("Data Handle"=w724, "Camera Handle"=w723) -> ("error out"=w726:errorcluster, "Data Handle"=w721:u32)  [unwired: 1 in, 1 out]
                        n198 = Unbundle(w685) -> (w693:u16[][], "XResAct"=w692:u16, "YResAct"=w691:u16, "BufNrOut"=w690:i16, "BufNrOut"=w689:i16, "ErrorOut"=w688:errorcluster, "hout"=w687:u64, "Bits/pixel"=w686:u16)
                        n199 = call <userlib>:"DisplayImage.vi"("error in"=w726, "Image Handle"=w721, "Display Handle"=w725) -> ()  [unwired: 1 in, 2 out]
                        n200 = call <userlib>:"ImageGetArrayI32.vi"("Image Handle"=w721) -> ("Array int 32"=w702:i32[][])  [unwired: 2 in, 2 out]
                        n201 = To Word Integer(number=w702) -> (16bit integer=w701:i16[][])
                        n202 = call "AddBufferEX.vi"("ph"=w687, "BuffNr"=i16 0, "1stImage"=w696, "LastImage"=w696, "error in (no error)"=w688, "XRes"=w692, "YRes"=w691, "BitPerPixel"=w686) -> ("hout"=w698:u64, "error out"=w697:errorcluster)  [unwired: 5 in, 1 out]
                        n203 = call "WaitForBuffer.vi"("ph"=w698, "sBufNr"=w689, "sBufNr 2"=w690, "timeout"=100, "error in (no error)"=w697) -> ("hout"=w700:u64)  [unwired: 10 in, 4 out]
                        n204 = call "GetImageBuffer2D.vi"("ph"=w700, "BuffIn"=w693, "BuffNr"=i16 0, "xRes"=w692, "yRes"=w691, "Bitresolution"=w686) -> ("BuffOut"=w684:u16[][])  [unwired: 6 in, 3 out]
                        n205 = Array Size(array=w684) -> (size(s)=w703:i32[])
                        n206 = Index Array(array=w703, index=0) -> (element=w708:i32)
                        n207 = Index Array(array=w703, index=1) -> (element=w707:i32)
                        n208 = To Word Integer(number=w708) -> (16bit integer=w709:i16)
                        n209 = To Word Integer(number=w707) -> (16bit integer=w706:i16)
                        n210 = Write to Binary File(file (use dialog)=w717, data=w709, 5:FALSE ("prepend array or string size? (T)"), 9:w710) -> (refnum out=w716:refnum<file>)  [unwired: 2 in, 2 out]
                        n211 = Write to Binary File(file (use dialog)=w716, data=w706, 5:FALSE ("prepend array or string size? (T)"), 9:w710) -> (refnum out=w715:refnum<file>)  [unwired: 2 in, 2 out]
                        n212 = To Word Integer(number=3 ("index")) -> (16bit integer=w705:i16)
                        n213 = Write to Binary File(file (use dialog)=w715, data=w705, 5:FALSE ("prepend array or string size? (T)"), 9:w710) -> (refnum out=w714:refnum<file>)  [unwired: 2 in, 2 out]
                        n214 = Write to Binary File(file (use dialog)=w714, data=w684, 5:FALSE ("prepend array or string size? (T)"), 9:w710) -> (error out=w720:errorcluster)  [unwired: 2 in, 2 out]
                      }
                      frame #2 {
                        n215 = Quotient & Remainder(x=w727, y=u32 10) -> (floor(x/y)=w728:u32)  [unwired: 1 out]
                        n216 = Add(x=w728, y=w727) -> (x+y=w730:u32)
                        n217 = Wait (ms)(milliseconds to wait=w730) -> ()  [unwired: 1 out]
                      }
                      frame #3 {
                        w743 = 0
                        n218 = call <userlib>:"CameraGetData.vi"("Data Handle"=w752, "Camera Handle"=w756) -> ("Data Handle"=w751:u32)  [unwired: 1 in, 2 out]
                        n219 = Unbundle(w732) -> (w740:u16[][], "XResAct"=w739:u16, "YResAct"=w738:u16, "BufNrOut"=w737:i16, "BufNrOut"=w736:i16, "ErrorOut"=w735:errorcluster, "hout"=w734:u64, "Bits/pixel"=w733:u16)
                        n220 = call <userlib>:"DisplayImage.vi"("Image Handle"=w751, "Display Handle"=w753) -> ()  [unwired: 2 in, 2 out]
                        n221 = call <userlib>:"ImageGetArrayI32.vi"("Image Handle"=w751) -> ("Array int 32"=w749:i32[][])  [unwired: 2 in, 2 out]
                        n222 = To Word Integer(number=w749) -> (16bit integer=w748:i16[][])
                        n223 = call "AddBufferEX.vi"("ph"=w734, "BuffNr"=i16 0, "1stImage"=w743, "LastImage"=w743, "error in (no error)"=w735, "XRes"=w739, "YRes"=w738, "BitPerPixel"=w733) -> ("hout"=w745:u64, "error out"=w744:errorcluster)  [unwired: 5 in, 1 out]
                        n224 = call "WaitForBuffer.vi"("ph"=w745, "sBufNr"=w736, "sBufNr 2"=w737, "timeout"=100, "error in (no error)"=w744) -> ("hout"=w747:u64)  [unwired: 10 in, 4 out]
                        n225 = call "GetImageBuffer2D.vi"("ph"=w747, "BuffIn"=w740, "BuffNr"=i16 0, "xRes"=w739, "yRes"=w738, "Bitresolution"=w733) -> ("BuffOut"=w731:u16[][])  [unwired: 6 in, 3 out]
                        n226 = Write to Binary File(file (use dialog)=w754, data=w731, 5:FALSE ("prepend array or string size? (T)"), 9:T5."little-endian" ("byte order (0:big-endian, network order)")) -> ()  [unwired: 2 in, 3 out]
                      }
                      frame #4 {
                        n227 = Quotient & Remainder(x=w757, y=u32 10) -> (floor(x/y)=w758:u32)  [unwired: 1 out]
                        n228 = Add(x=w758, y=w757) -> (x+y=w760:u32)
                        n229 = Wait (ms)(milliseconds to wait=w760) -> ()  [unwired: 1 out]
                      }
                      frame #5 {
                        w773 = 0
                        n230 = call <userlib>:"CameraGetData.vi"("Data Handle"=w782, "Camera Handle"=w786) -> ("Data Handle"=w781:u32)  [unwired: 1 in, 2 out]
                        n231 = Unbundle(w762) -> (w770:u16[][], "XResAct"=w769:u16, "YResAct"=w768:u16, "BufNrOut"=w767:i16, "BufNrOut"=w766:i16, "ErrorOut"=w765:errorcluster, "hout"=w764:u64, "Bits/pixel"=w763:u16)
                        n232 = call <userlib>:"DisplayImage.vi"("Image Handle"=w781, "Display Handle"=w783) -> ()  [unwired: 2 in, 2 out]
                        n233 = call <userlib>:"ImageGetArrayI32.vi"("Image Handle"=w781) -> ("Array int 32"=w779:i32[][])  [unwired: 2 in, 2 out]
                        n234 = To Word Integer(number=w779) -> (16bit integer=w778:i16[][])
                        n235 = call "AddBufferEX.vi"("ph"=w764, "BuffNr"=i16 0, "1stImage"=w773, "LastImage"=w773, "error in (no error)"=w765, "XRes"=w769, "YRes"=w768, "BitPerPixel"=w763) -> ("hout"=w775:u64, "error out"=w774:errorcluster)  [unwired: 5 in, 1 out]
                        n236 = call "WaitForBuffer.vi"("ph"=w775, "sBufNr"=w766, "sBufNr 2"=w767, "timeout"=100, "error in (no error)"=w774) -> ("hout"=w777:u64)  [unwired: 10 in, 4 out]
                        n237 = call "GetImageBuffer2D.vi"("ph"=w777, "BuffIn"=w770, "BuffNr"=i16 0, "xRes"=w769, "yRes"=w768, "Bitresolution"=w763) -> ("BuffOut"=w761:u16[][])  [unwired: 6 in, 3 out]
                        n238 = Write to Binary File(file (use dialog)=w784, data=w761, 5:FALSE ("prepend array or string size? (T)"), 9:T5."little-endian" ("byte order (0:big-endian, network order)")) -> ()  [unwired: 2 in, 3 out]
                      }
                      frame #6 {
                        # "Indicate DB\nIssue"
                        # "Number of replacements is number of lines"
                        n239 = Search and Replace String(replace all?=TRUE ("replace all? (F)"), input string=w790, search string="(") -> (result string=w799:string)  [unwired: 5 in, 3 out]
                        n240 = Search and Replace String(replace all?=TRUE ("replace all? (F)"), input string=w799, search string=")") -> (result string=w787:string, number of replacements=w788:i32)  [unwired: 5 in, 2 out]
                        n241 = local write "Database Output"(w787) -> ()
                        n242 = for {
                          N: w788 -> [_]
                          tunnel: w787 -> [w824]
                          tunnel: w795 -> [w820]
                          i -> [w825]
                          w812 = T5."little-endian" ("byte order (0:big-endian, network order)")
                          n243 = Pick Line(multi-line string=w824, line index=w825) -> (output string=w823:string)  [unwired: 1 in]
                          n244 = Match Pattern(string=w823, regular expression="\\s") -> (before substring=w815:string, after substring=w821:string)  [unwired: 1 in, 2 out]
                          n245 = Concatenate Strings(w815) -> (w814:string)
                          n246 = Fract/Exp String To Number(string=w821) -> (number=w809:dbl)  [unwired: 3 in, 1 out]
                          n247 = To Double Precision Float(number=w809) -> (double precision float=w807:dbl)
                          n248 = Write to Binary File(file (use dialog)=w820, data=w814, 5:FALSE ("prepend array or string size? (T)"), 9:w812) -> (refnum out=w816:refnum<file>, error out=w817:errorcluster)  [unwired: 2 in, 1 out]
                          n249 = To Byte Integer(number=0) -> (8bit integer=w806:i8)
                          n250 = Write to Binary File(file (use dialog)=w816, data=w806, error in=w817, 5:FALSE ("prepend array or string size? (T)"), 9:T5."little-endian" ("byte order (0:big-endian, network order)")) -> (refnum out=w810:refnum<file>, error out=w813:errorcluster)  [unwired: 1 in, 1 out]
                          n251 = Write to Binary File(file (use dialog)=w810, data=w807, error in=w813, 5:FALSE ("prepend array or string size? (T)"), 9:w812) -> ()  [unwired: 1 in, 3 out]
                        }
                        n252 = String Length(string=w787) -> (length=w789:i32)
                        n253 = Greater?(x=w789, y=10) -> (0:w791:bool)
                        n254 = case shown="False" w791 {
                          tunnel: w788 -> [w801 w803]
                          frame False {
                            n255 = local write "Entries in DB String"(w801) -> ()
                            n256 = local write "Database OK?"(TRUE ("Database OK?")) -> ()
                          }
                          frame True {
                            n257 = local write "Entries in DB String"(w803) -> ()
                            n258 = local write "Database OK?"(FALSE ("Database OK?")) -> ()
                          }
                        }
                        n259 = shared-variable-write(refnum<k21> "ni.var.psp://my computer/Untitled Library 1/CSHQ_1_Time" ("shared variable refnum in"), w793) -> ()  [unwired: 1 in, 2 out]
                      }
                      frame #7 {
                        n260 = Close File(refnum=w826) -> ()  [unwired: 1 in, 2 out]
                      }
                    }
                    n261 = local read "PF Scale"() -> (w654:dbl)
                    n262 = Reshape Array(w644, 1447680 ("dimension size")) -> (w650:u16[])
                    n263 = Reshape Array(w643, 1447680 ("dimension size")) -> (w648:u16[])
                    n264 = Reshape Array(w642, 1447680 ("dimension size")) -> (w649:u16[])
                    n265 = shared-variable "My Computer\\DASLib.lvlib\\CSHQ_Atoms"(w650) -> (error out=w647:errorcluster)  [unwired: 1 in]
                    n266 = shared-variable "My Computer\\DASLib.lvlib\\CSHQ_Bright"(w648, error in=w647) -> (error out=w646:errorcluster)
                    n267 = shared-variable "My Computer\\DASLib.lvlib\\CSHQ_Dark"(w649, error in=w646) -> (error out=w645:errorcluster)
                  }
                  frame 0 {
                    # "DEFAULT: Send CoolSnap to DER"
                    # "This stacked sequence builds the .AIA file"
                    n268 = stacked-sequence {
                      tunnel: w851 -> [_ w879 _ w909 _ w936 _ _]
                      tunnel: w850 -> [_ _ _ _ _ _ _ _]
                      tunnel: w849 -> [_ w881 _ w908 _ w935 _ _]
                      tunnel: w848 -> [_ w880 _ w907 _ w934 _ _]
                      tunnel: w847 -> [_ _ w883 _ w910 _ _ _]
                      tunnel: [_ w871 _ _ _ _ _ _] -> w830
                      tunnel: [_ _ _ w904 _ _ _ _] -> w829
                      tunnel: [_ _ _ _ _ w931 _ _] -> w827
                      tunnel: w846 -> [_ w855 _ w888 _ w915 _ _]
                      tunnel: [_ w854 _ _ _ _ _ _] -> w845
                      tunnel: [_ _ _ w887 _ _ _ _] -> w844
                      tunnel: [_ _ _ _ _ w914 _ _] -> w828
                      tunnel: w843 -> [_ _ _ _ _ _ w942 _]
                      tunnel: w842 -> [_ _ _ _ _ _ w938 _]
                      tunnel: [_ w853 _ _ _ _ _ _] -> w841
                      frame #0 {
                        # "NOT saving, so do nothing here."
                      }
                      frame #1 {
                        w866 = 0
                        (unwired) T5."little-endian" ("byte order (0:big-endian, network order)")
                        n269 = call <userlib>:"CameraGetData.vi"("Data Handle"=w880, "Camera Handle"=w879) -> ("error out"=w882:errorcluster, "Data Handle"=w878:u32)  [unwired: 1 in, 1 out]
                        n270 = Unbundle(w855) -> (w863:u16[][], "XResAct"=w862:u16, "YResAct"=w861:u16, "BufNrOut"=w860:i16, "BufNrOut"=w859:i16, "ErrorOut"=w858:errorcluster, "hout"=w857:u64, "Bits/pixel"=w856:u16)
                        n271 = call <userlib>:"DisplayImage.vi"("error in"=w882, "Image Handle"=w878, "Display Handle"=w881) -> ()  [unwired: 1 in, 2 out]
                        n272 = call <userlib>:"ImageGetArrayI32.vi"("Image Handle"=w878) -> ("Array int 32"=w872:i32[][])  [unwired: 2 in, 2 out]
                        n273 = To Word Integer(number=w872) -> (16bit integer=w871:i16[][])
                        n274 = Array Size(array=w872) -> (size(s)=w873:i32[])
                        n275 = call "AddBufferEX.vi"("ph"=w857, "BuffNr"=i16 0, "1stImage"=w866, "LastImage"=w866, "error in (no error)"=w858, "XRes"=w862, "YRes"=w861, "BitPerPixel"=w856) -> ("hout"=w868:u64, "error out"=w867:errorcluster)  [unwired: 5 in, 1 out]
                        n276 = Index Array(array=w873, index=0) -> (element=w875:i32)
                        n277 = Index Array(array=w873, index=1) -> (element=w874:i32)
                        n278 = To Word Integer(number=w875) -> ()  [unwired: 1 out]
                        n279 = To Word Integer(number=w874) -> ()  [unwired: 1 out]
                        n280 = call "WaitForBuffer.vi"("ph"=w868, "sBufNr"=w859, "sBufNr 2"=w860, "timeout"=100, "error in (no error)"=w867) -> ("hout"=w870:u64, "error out"=w852:errorcluster)  [unwired: 10 in, 3 out]
                        n281 = call "GetImageBuffer2D.vi"("ph"=w870, "BuffIn"=w863, "BuffNr"=i16 0, "error in (no error)"=w852, "xRes"=w862, "yRes"=w861, "Bitresolution"=w856) -> ("BuffOut"=w854:u16[][], "error out"=w853:errorcluster)  [unwired: 5 in, 2 out]
                      }
                      frame #2 {
                        n282 = Quotient & Remainder(x=w883, y=u32 10) -> (floor(x/y)=w884:u32)  [unwired: 1 out]
                        n283 = Add(x=w884, y=w883) -> (x+y=w886:u32)
                        n284 = Wait (ms)(milliseconds to wait=w886) -> ()  [unwired: 1 out]
                      }
                      frame #3 {
                        w899 = 0
                        (unwired) T5."little-endian" ("byte order (0:big-endian, network order)")
                        (unwired) FALSE ("prepend array or string size? (T)")
                        n285 = call <userlib>:"CameraGetData.vi"("Data Handle"=w907, "Camera Handle"=w909) -> ("Data Handle"=w906:u32)  [unwired: 1 in, 2 out]
                        n286 = Unbundle(w888) -> (w896:u16[][], "XResAct"=w895:u16, "YResAct"=w894:u16, "BufNrOut"=w893:i16, "BufNrOut"=w892:i16, "ErrorOut"=w891:errorcluster, "hout"=w890:u64, "Bits/pixel"=w889:u16)
                        n287 = call <userlib>:"DisplayImage.vi"("Image Handle"=w906, "Display Handle"=w908) -> ()  [unwired: 2 in, 2 out]
                        n288 = call <userlib>:"ImageGetArrayI32.vi"("Image Handle"=w906) -> ("Array int 32"=w905:i32[][])  [unwired: 2 in, 2 out]
                        n289 = To Word Integer(number=w905) -> (16bit integer=w904:i16[][])
                        n290 = call "AddBufferEX.vi"("ph"=w890, "BuffNr"=i16 0, "1stImage"=w899, "LastImage"=w899, "error in (no error)"=w891, "XRes"=w895, "YRes"=w894, "BitPerPixel"=w889) -> ("hout"=w901:u64, "error out"=w900:errorcluster)  [unwired: 5 in, 1 out]
                        n291 = call "WaitForBuffer.vi"("ph"=w901, "sBufNr"=w892, "sBufNr 2"=w893, "timeout"=100, "error in (no error)"=w900) -> ("hout"=w903:u64)  [unwired: 10 in, 4 out]
                        n292 = call "GetImageBuffer2D.vi"("ph"=w903, "BuffIn"=w896, "BuffNr"=i16 0, "xRes"=w895, "yRes"=w894, "Bitresolution"=w889) -> ("BuffOut"=w887:u16[][])  [unwired: 6 in, 3 out]
                      }
                      frame #4 {
                        n293 = Quotient & Remainder(x=w910, y=u32 10) -> (floor(x/y)=w911:u32)  [unwired: 1 out]
                        n294 = Add(x=w911, y=w910) -> (x+y=w913:u32)
                        n295 = Wait (ms)(milliseconds to wait=w913) -> ()  [unwired: 1 out]
                      }
                      frame #5 {
                        w926 = 0
                        (unwired) T5."little-endian" ("byte order (0:big-endian, network order)")
                        (unwired) FALSE ("prepend array or string size? (T)")
                        n296 = call <userlib>:"CameraGetData.vi"("Data Handle"=w934, "Camera Handle"=w936) -> ("Data Handle"=w933:u32)  [unwired: 1 in, 2 out]
                        n297 = Unbundle(w915) -> (w923:u16[][], "XResAct"=w922:u16, "YResAct"=w921:u16, "BufNrOut"=w920:i16, "BufNrOut"=w919:i16, "ErrorOut"=w918:errorcluster, "hout"=w917:u64, "Bits/pixel"=w916:u16)
                        n298 = call <userlib>:"DisplayImage.vi"("Image Handle"=w933, "Display Handle"=w935) -> ()  [unwired: 2 in, 2 out]
                        n299 = call <userlib>:"ImageGetArrayI32.vi"("Image Handle"=w933) -> ("Array int 32"=w932:i32[][])  [unwired: 2 in, 2 out]
                        n300 = To Word Integer(number=w932) -> (16bit integer=w931:i16[][])
                        n301 = call "AddBufferEX.vi"("ph"=w917, "BuffNr"=i16 0, "1stImage"=w926, "LastImage"=w926, "error in (no error)"=w918, "XRes"=w922, "YRes"=w921, "BitPerPixel"=w916) -> ("hout"=w928:u64, "error out"=w927:errorcluster)  [unwired: 5 in, 1 out]
                        n302 = call "WaitForBuffer.vi"("ph"=w928, "sBufNr"=w919, "sBufNr 2"=w920, "timeout"=100, "error in (no error)"=w927) -> ("hout"=w930:u64)  [unwired: 10 in, 4 out]
                        n303 = call "GetImageBuffer2D.vi"("ph"=w930, "BuffIn"=w923, "BuffNr"=i16 0, "xRes"=w922, "yRes"=w921, "Bitresolution"=w916) -> ("BuffOut"=w914:u16[][])  [unwired: 6 in, 3 out]
                      }
                      frame #6 {
                        # "Indicate DB\nIssue"
                        # "Number of replacements is number of lines"
                        n304 = Search and Replace String(replace all?=TRUE ("replace all? (F)"), input string=w938, search string="(") -> (result string=w947:string)  [unwired: 5 in, 3 out]
                        n305 = Search and Replace String(replace all?=TRUE ("replace all? (F)"), input string=w947, search string=")") -> (result string=w941:string)  [unwired: 5 in, 3 out]
                        n306 = String Length(string=w941) -> (length=w937:i32)
                        n307 = Greater?(x=w937, y=10) -> (0:w939:bool)
                        n308 = case shown="False" w939 {
                          tunnel: w937 -> [w949 w951]
                          frame False {
                            n309 = local write "Entries in DB String"(w949) -> ()
                            n310 = local write "Database OK?"(TRUE ("Database OK?")) -> ()
                          }
                          frame True {
                            n311 = local write "Entries in DB String"(w951) -> ()
                          }
                        }
                        n312 = shared-variable-write(refnum<k21> "ni.var.psp://my computer/Untitled Library 1/CSHQ_1_Time" ("shared variable refnum in"), w942) -> ()  [unwired: 1 in, 2 out]
                      }
                      frame #7 {
                      }
                    }
                    n313 = local read "PF Scale"() -> (w840:dbl)
                    n314 = Reshape Array(w830, 1447680 ("dimension size")) -> (w835:i16[])
                    n315 = Reshape Array(w829, 1447680 ("dimension size")) -> (w833:i16[])
                    n316 = Reshape Array(w827, 1447680 ("dimension size")) -> (w834:i16[])
                    n317 = shared-variable "My Computer\\DASLib.lvlib\\CSHQ_Atoms"(w835) -> (error out=w832:errorcluster)  [unwired: 1 in]
                    n318 = shared-variable "My Computer\\DASLib.lvlib\\CSHQ_Bright"(w833, error in=w832) -> (error out=w831:errorcluster)
                    n319 = shared-variable "My Computer\\DASLib.lvlib\\CSHQ_Dark"(w834, error in=w831) -> ()  [unwired: 1 out]
                  }
                }
                n320 = shared-variable-write(refnum<k21> "ni.var.psp://my computer/Untitled Library 1/CSHQ_1_Changed" ("shared variable refnum in"), TRUE) -> ()  [unwired: 1 in, 2 out]
                n321 = Subtract(x=w395, y=w392) -> (x-y=w446:i16[][])
                n322 = Subtract(x=w394, y=w392) -> (x-y=w445:i16[][])
                n323 = Subtract(x=w432, y=w422) -> (x-y=w425:i32[][])
                n324 = Subtract(x=w435, y=w422) -> (x-y=w423:i32[][])
                n325 = for {
                  N -> [w984]
                  shift-right: [w985] -> w431
                  shift-left: w432 -> [w987]
                  tunnel: w432 -> [w986] mode=indexing
                  i -> [w980]
                  n326 = Subtract(x=w984, y=1) -> (x-y=w982:i32)
                  n327 = Subtract(x=w982, y=w980) -> (x-y=w981:i32)
                  n328 = Replace Array Subset(array=w987, new element=w986, index (row)=w981) -> (w985:u16[][])  [unwired: 1 in]
                }
                n329 = for {
                  N -> [w976]
                  shift-right: [w977] -> w428
                  shift-left: w429 -> [w979]
                  tunnel: w429 -> [w978] mode=indexing
                  i -> [w972]
                  n330 = Subtract(x=w976, y=1) -> (x-y=w974:i32)
                  n331 = Subtract(x=w974, y=w972) -> (x-y=w973:i32)
                  n332 = Replace Array Subset(array=w979, new element=w978, index (row)=w973) -> (w977:u16[][])  [unwired: 1 in]
                }
                n333 = for {
                  N -> [w992]
                  shift-right: [w993] -> w434
                  shift-left: w435 -> [w995]
                  tunnel: w435 -> [w994] mode=indexing
                  i -> [w988]
                  n334 = Subtract(x=w992, y=1) -> (x-y=w990:i32)
                  n335 = Subtract(x=w990, y=w988) -> (x-y=w989:i32)
                  n336 = Replace Array Subset(array=w995, new element=w994, index (row)=w989) -> (w993:u16[][])  [unwired: 1 in]
                }
                n337 = for {
                  N -> [w1008]
                  shift-right: [w1009] -> w436
                  shift-left: w394 -> [w1011]
                  tunnel: w394 -> [w1010] mode=indexing
                  i -> [w1004]
                  n338 = Subtract(x=w1008, y=1) -> (x-y=w1006:i32)
                  n339 = Subtract(x=w1006, y=w1004) -> (x-y=w1005:i32)
                  n340 = Replace Array Subset(array=w1011, new element=w1010, index (row)=w1005) -> (w1009:i16[][])  [unwired: 1 in]
                }
                n341 = for {
                  N -> [w1016]
                  shift-right: [w1017] -> w437
                  shift-left: w395 -> [w1019]
                  tunnel: w395 -> [w1018] mode=indexing
                  i -> [w1012]
                  n342 = Subtract(x=w1016, y=1) -> (x-y=w1014:i32)
                  n343 = Subtract(x=w1014, y=w1012) -> (x-y=w1013:i32)
                  n344 = Replace Array Subset(array=w1019, new element=w1018, index (row)=w1013) -> (w1017:i16[][])  [unwired: 1 in]
                }
                n345 = for {
                  N -> [w1000]
                  shift-right: [w1001] -> w409
                  shift-left: w392 -> [w1003]
                  tunnel: w392 -> [w1002] mode=indexing
                  i -> [w996]
                  n346 = Subtract(x=w1000, y=1) -> (x-y=w998:i32)
                  n347 = Subtract(x=w998, y=w996) -> (x-y=w997:i32)
                  n348 = Replace Array Subset(array=w1003, new element=w1002, index (row)=w997) -> (w1001:i16[][])  [unwired: 1 in]
                }
                n349 = Multiply(x=w425, y=w426) -> (x*y=w424:dbl[][])
                n350 = Multiply(x=w445, y="Scaling") -> (x*y=w444:dbl[][])
                n351 = Divide(x=w423, y=w424) -> (x/y=w438:dbl[][])
                n352 = Divide(x=w446, y=w444) -> (x/y=w443:dbl[][])
                n353 = for {
                  N -> [w1025]
                  shift-right: [w1026] -> w439
                  shift-left: w438 -> [w1027]
                  tunnel: w438 -> [w1020] mode=indexing
                  i -> [w1021]
                  n354 = Subtract(x=w1025, y=1) -> (x-y=w1023:i32)
                  n355 = Subtract(x=w1023, y=w1021) -> (x-y=w1022:i32)
                  n356 = Replace Array Subset(array=w1027, new element=w1020, index (row)=w1022) -> (w1026:dbl[][])  [unwired: 1 in]
                }
                n357 = Array Size(array=w443) -> ()  [unwired: 1 out]
                n358 = for {
                  N -> [w1032]
                  shift-right: [w1033] -> w405
                  shift-left: w443 -> [w1035]
                  tunnel: w443 -> [w1034] mode=indexing
                  i -> [w1028]
                  n359 = Subtract(x=w1032, y=1) -> (x-y=w1030:i32)
                  n360 = Subtract(x=w1030, y=w1028) -> (x-y=w1029:i32)
                  n361 = Replace Array Subset(array=w1035, new element=w1034, index (row)=w1029) -> (w1033:dbl[][])  [unwired: 1 in]
                }
                n362 = Transpose 2D Array(2D array=w409) -> (transposed array=→"Dark Field":i16[][])
                n363 = Transpose 2D Array(2D array=w431) -> (transposed array=→"PF No Atoms":u16[][])
                n364 = Transpose 2D Array(2D array=w428) -> (transposed array=→"PF Dark":u16[][])
                n365 = Transpose 2D Array(2D array=w434) -> (transposed array=→"PF Atoms":u16[][])
                n366 = Transpose 2D Array(2D array=w437) -> (transposed array=→"Atoms":i16[][])
                n367 = Transpose 2D Array(2D array=w436) -> (transposed array=→"No Atoms":i16[][])
                n368 = Transpose 2D Array(2D array=w439) -> (transposed array=→"Intensity Graph":dbl[][])
                n369 = Transpose 2D Array(2D array=w405) -> (transposed array=w406:dbl[][])
                n370 = case shown="False" w419 {
                  tunnel: w406 -> [w956 w971]
                  tunnel: w417 -> [w960 w970]
                  tunnel: [w952 w969] -> w416
                  frame False {
                    n371 = Flush Queue(queue=w960) -> (queue out=w958:refnum<queue>, remaining elements=w959:cluster{"Normalized Image":dbl[][]}[])  [unwired: 1 in, 1 out]
                    n372 = for {
                      tunnel: w959 -> [w968] mode=indexing
                      tunnel: w958 -> [w966]
                      tunnel: [w965] -> w957
                      n373 = Unbundle By Name(w968) -> ("Normalized Image"=w967:dbl[][])
                      n374 = Enqueue Element At Opposite End(queue=w966, element=w967) -> (queue out=w965:refnum<queue>)  [unwired: 2 in, 2 out]
                    }
                    n375 = Lossy Enqueue Element(queue=w957, element=w956) -> (queue out=w955:refnum<queue>)  [unwired: 1 in, 3 out]
                    n376 = Flush Queue(queue=w955) -> (queue out=w954:refnum<queue>, remaining elements=w953:cluster{"Normalized Image":dbl[][]}[])  [unwired: 1 in, 1 out]
                    n377 = for {
                      tunnel: w953 -> [w964] mode=indexing
                      tunnel: w954 -> [w962]
                      tunnel: [w961] -> w952
                      n378 = Unbundle By Name(w964) -> ("Normalized Image"=w963:dbl[][])
                      n379 = Enqueue Element At Opposite End(queue=w962, element=w963) -> (queue out=w961:refnum<queue>)  [unwired: 2 in, 2 out]
                    }
                  }
                  frame True {
                    n380 = Enqueue Element At Opposite End(queue=w970, element=w971) -> (queue out=w969:refnum<queue>)  [unwired: 2 in, 2 out]
                  }
                }
                n381 = call "DBStringToAssociativeArray.vi"("Raw DB String"=w399) -> ("Values"=w397:dbl[], "Names"=w398:string[])  [unwired: 9 in]
                n382 = Reshape Array(w395, 1447680 ("dimension size")) -> ()  [unwired: 1 out]
                n383 = Reshape Array(w394, 1447680 ("dimension size")) -> ()  [unwired: 1 out]
                n384 = Reshape Array(w392, 1447680 ("dimension size")) -> ()  [unwired: 1 out]
                n385 = shared-variable "My Computer\\DASLib.lvlib\\CiceroVariableNames"(w398, error in=w391) -> (error out=w390:errorcluster)
                n386 = shared-variable "My Computer\\DASLib.lvlib\\CiceroVariableValues"(w397, error in=w390) -> (error out=w389:errorcluster)
                n387 = shared-variable "My Computer\\DASLib.lvlib\\UpdateFlag"(TRUE ("UpdateFlag"), error in=w389) -> ()  [unwired: 1 out]
              }
            }
            n388 = Add(x=-1.54, y=w245) -> (x+y=→"Top of Chamber Monitor":dynamicdata)
            n389 = shared-variable-read(refnum<k21> "ni.var.psp://my computer/Untitled Library 1/CSHQ_1_Changed" ("shared variable refnum in"), TRUE) -> (w259:refnum<k21>, w252:bool)  [unwired: 1 in, 2 out]
            n390 = Get Queue Status(queue=w250) -> (queue out=w262:refnum<queue>, # elements in queue=w258:i32)  [unwired: 2 in, 6 out]
            n391 = case shown="True" w252 {
              tunnel: w259 -> [_ _]
              tunnel: w258 -> [_ w329]
              tunnel: w257 -> [w317 w330]
              tunnel: [w317 w328] -> w256
              tunnel: [TRUE w325] -> _
              tunnel: w250 -> [_ w319]
              frame False {
              }
              frame True {
                w325 = FALSE
                n392 = Get Queue Status(queue=w319) -> (queue out=w318:refnum<queue>, # elements in queue=w324:i32)  [unwired: 2 in, 6 out]
                n393 = Less?(x=w329, y=5) -> (x < y?=w331:bool)
                n394 = Wait (ms)(milliseconds to wait=u32 150) -> ()  [unwired: 1 out]
                n395 = case shown="True" w331 {
                  tunnel: w330 -> [w347 w382]
                  tunnel: w329 -> [_ w379]
                  tunnel: [w345 w380] -> w328
                  tunnel: [w344 w377] -> w320
                  frame False {
                    n396 = for {
                      N: 5 -> [_]
                      tunnel: w347 -> [w352]
                      shift-right: [w350] -> w345
                      shift-left: _ -> [w349]
                      tunnel: [w348] -> w344
                      i -> [w351]
                      w348 = 4.0 ("Value")
                      n397 = property on="Display Image" class="Ring (strict)"("Value"=w348) -> ()  [unwired: 2 in, 2 out]
                      n398 = case shown="1..3" w351 {
                        selector: w351 -> [_ w361 w371]
                        tunnel: w352 -> [_ w362 w376]
                        tunnel: [cluster{"date/time string":string, i32}[] [] w360 w368] -> w350
                        tunnel: w349 -> [_ w359 w375]
                        frame 0, Default {
                        }
                        frame 1..3 {
                          n399 = Index Array(array=w362, index=w361) -> (element=w358:cluster{"date/time string":string, i32})
                          n400 = Unbundle(w358) -> ("date/time string"=w357:string, w356:i32)
                          n401 = Decrement(x=w356) -> (x-1=w355:i32)
                          n402 = Bundle("date/time string"=w357, w355) -> (w354:cluster{"date/time string":string, i32})  [unwired: 1 in]
                          n403 = Build Array (concatenate)(w359, w354) -> (w360:cluster{"date/time string":string, i32}[])
                        }
                        frame 4 {
                          n404 = Index Array(array=w376, index=w371) -> (element=w364:cluster{"date/time string":string, i32})
                          n405 = Unbundle(w364) -> ("date/time string"=w367:string, w366:i32)
                          n406 = Decrement(x=w366) -> (x-1=w365:i32)
                          n407 = Bundle("date/time string"=w367, w365) -> (w363:cluster{"date/time string":string, i32})  [unwired: 1 in]
                          n408 = Build Array (concatenate)(w375, w363) -> (w372:cluster{"date/time string":string, i32}[])
                          n409 = shared-variable-read(refnum<k21> "ni.var.psp://my computer/Untitled Library 1/CSHQ_1_Time" ("shared variable refnum in"), "bullshit" ("search string")) -> (w370:string)  [unwired: 1 in, 3 out]
                          n410 = Bundle("search string"=w370, w371) -> (w369:cluster{"search string":string, i32})  [unwired: 1 in]
                          n411 = Build Array (concatenate)(w372, w369) -> (w368:cluster{"search string":string, i32}[])
                        }
                      }
                    }
                  }
                  frame True {
                    n412 = Subtract(x=w379, y=1) -> (x-y=w377:i32)
                    n413 = property on="Display Image" class="Ring (strict)"("Value"=w377) -> ()  [unwired: 2 in, 2 out]
                    n414 = shared-variable-read(refnum<k21> "ni.var.psp://my computer/Untitled Library 1/CSHQ_1_Time" ("shared variable refnum in"), "string" ("search string")) -> (w383:string)  [unwired: 1 in, 3 out]
                    n415 = Bundle("search string"=w383, w377) -> (w381:cluster{"search string":string, i32})  [unwired: 1 in]
                    n416 = Build Array (concatenate)(w382, w381) -> (w380:cluster{"search string":string, i32}[])
                  }
                }
                n417 = Flush Queue(queue=w318) -> (queue out=w322:refnum<queue>, remaining elements=w323:cluster{"Normalized Image":dbl[][]}[])  [unwired: 1 in, 1 out]
                n418 = shared-variable-write(refnum<k21> "ni.var.psp://my computer/Untitled Library 1/CSHQ_1_Changed" ("shared variable refnum in"), w325) -> ()  [unwired: 1 in, 2 out]
                n419 = To Word Integer(number=w320) -> (16bit integer=w321:i16)
                n420 = for {
                  tunnel: w323 -> [w342] mode=indexing
                  tunnel: w322 -> [w341]
                  tunnel: [w340] -> _
                  tunnel: w321 -> [w334]
                  tunnel: w324 -> [w335]
                  i -> [w339]
                  n421 = Unbundle By Name(w342) -> ("Normalized Image"=w336:dbl[][])
                  n422 = Increment(x=w334) -> (x+1=w333:i16)
                  n423 = Subtract(x=w335, y=w333) -> (x-y=w338:i32)
                  n424 = Enqueue Element(queue=w341, element=w336) -> (queue out=w340:refnum<queue>)  [unwired: 2 in, 2 out]
                  n425 = Equal?(x=w338, y=w339) -> (x = y?=w337:bool)
                  n426 = case shown="True" w337 {
                    tunnel: w336 -> [_ w343]
                    frame False {
                    }
                    frame True {
                      n427 = local write "Normalized Image"(w343) -> ()
                    }
                  }
                }
              }
            }
            n428 = Greater?(x=w258, y=0) -> (0:w254:bool)
            n429 = event shown="[0] \"Display Image\": Value Change" {
              selector: _ -> [_ _]
              dyn-events: _ -> [_ _]
              timeout: 1 -> [_ _]
              tunnel: [w295 w315] -> w263
              tunnel: w262 -> [w294 w315]
              tunnel: w258 -> [w293 _]
              tunnel: w254 -> [w292 _]
              tunnel: "Display Image" -> [w291 _]
              event "Display Image": Value Change {
                n430 = event-data() -> ()  [unwired: 1 in, 5 out]
                n431 = case shown="True" w292 {
                  tunnel: [w296 w301] -> w295
                  tunnel: w294 -> [w296 w299]
                  tunnel: w293 -> [_ w298]
                  tunnel: w291 -> [_ w297]
                  frame False {
                  }
                  frame True {
                    n432 = To Word Integer(number=w297) -> (16bit integer=w300:i16)
                    n433 = Flush Queue(queue=w299) -> (queue out=w302:refnum<queue>, remaining elements=w303:cluster{"Normalized Image":dbl[][]}[])  [unwired: 1 in, 1 out]
                    n434 = for {
                      tunnel: w303 -> [w313] mode=indexing
                      tunnel: w302 -> [w312]
                      tunnel: [w311] -> w301
                      tunnel: w300 -> [w305]
                      tunnel: w298 -> [w306]
                      i -> [w310]
                      n435 = Unbundle By Name(w313) -> ("Normalized Image"=w307:dbl[][])
                      n436 = Increment(x=w305) -> (x+1=w304:i16)
                      n437 = Subtract(x=w306, y=w304) -> (x-y=w309:i32)
                      n438 = Enqueue Element(queue=w312, element=w307) -> (queue out=w311:refnum<queue>)  [unwired: 2 in, 2 out]
                      n439 = Equal?(x=w309, y=w310) -> (x = y?=w308:bool)
                      n440 = case shown="True" w308 {
                        tunnel: w307 -> [_ w314]
                        frame False {
                        }
                        frame True {
                          "Normalized Image" <- w314
                        }
                      }
                    }
                  }
                }
              }
              event Timeout {
                n441 = event-data() -> ()  [unwired: 1 in, 2 out]
              }
            }
            n442 = property on="Display Image" class="Ring (strict)"("StringsAndValues[]"=w256) -> ()  [unwired: 2 in, 2 out]
          }
        }
        frame 2 {
          (unwired) cluster{"date/time string":string, i32}[] []
          n443 = Unbundle(w1047) -> ("Camera Handle"=w1046:u32, "File Handle"=w1050:u32, "Display Handle"=w1049:u32, "Image Handle"=w1048:u32)
          n444 = while {
            tunnel: "error in (no error) 3" -> [w1106]
            tunnel: w1046 -> [w1105]
            tunnel: [w1103] -> _
            tunnel: w1050 -> [_]
            tunnel: w1049 -> [w1102]
            tunnel: w1048 -> [w1101]
            tunnel: [w1079] -> _
            tunnel: w1045 -> [w1094]
            tunnel: w1044 -> [w1091]
            tunnel: w1043 -> [w1090]
            tunnel: w1042 -> [w1089]
            tunnel: w1041 -> [w1087]
            tunnel: w1040 -> [w1088]
            tunnel: w1039 -> [w1083]
            tunnel: w1038 -> [w1086]
            tunnel: w1037 -> [w1085]
            tunnel: [w1083] -> w1036
            stop <- w1093 continue-if-true
            w1072 = 0
            (unwired) 1
            # "Press and HOLD stop button to exit this loop."
            # "Stop Button"
            # "This loop simply grabs frames continuously from the two cameras."
            # "Shot 2: W/O Atoms"
            # "NI Scope"
            # "CoolSnap Camera Functions"
            # "ADC Inputs"
            n445 = Bundle(w1091, "XResAct"=w1090, "YResAct"=w1089, "BufNrOut"=w1088, "BufNrOut"=w1087, "ErrorOut"=w1086, "hout"=w1083, "Bits/pixel"=w1085) -> (w1084:T10)  [unwired: 1 in]
            n446 = call <userlib>:"CameraCheckData.vi"("Camera Handle"=w1105, "error in"=w1106) -> ("Camera Handle"=w1104:u32, "Number Of Frames Available"=w1099:i32)  [unwired: 1 out]
            n447 = Wait Until Next ms Multiple(millisecond multiple=1) -> (millisecond timer value=w1079:u32)
            n448 = control-ref of="?"() -> (w1055:refnum<vi>)
            n449 = Greater Or Equal?(x=w1099, y=1) -> ()  [unwired: 1 out]
            n450 = Unbundle(w1084) -> (w1069:u16[][], "XResAct"=w1068:u16, "YResAct"=w1067:u16, "BufNrOut"=w1066:i16, "BufNrOut"=w1065:i16, "ErrorOut"=w1064:errorcluster, "hout"=w1063:u64, "Bits/pixel"=w1062:u16)
            n451 = property class="Bool (strict)"(reference=w1055) -> ("Value"=w1054:bool)  [unwired: 1 in, 2 out]
            n452 = call "DAQ Assistant2"() -> ("data"=w1082:dynamicdata)  [unwired: 17 in, 2 out]
            n453 = call <userlib>:"CameraGetData.vi"("Data Handle"=w1101, "Camera Handle"=w1104) -> ("error out"=w1078:errorcluster, "Data Handle"=w1077:u32)  [unwired: 1 in, 1 out]
            n454 = Not(x=w1054) -> (.not. x?=w1092:bool)
            n455 = call <userlib>:"DisplayImage.vi"("error in"=w1078, "Image Handle"=w1077, "Display Handle"=w1102) -> ()  [unwired: 1 in, 2 out]
            n456 = call "AddBufferEX.vi"("ph"=w1063, "BuffNr"=i16 0, "1stImage"=w1072, "LastImage"=w1072, "error in (no error)"=w1064, "XRes"=w1068, "YRes"=w1067, "BitPerPixel"=w1062) -> ("hout"=w1074:u64, "error out"=w1073:errorcluster)  [unwired: 5 in, 1 out]
            n457 = call <userlib>:"ImageGetArrayI32.vi"("Image Handle"=w1077) -> ("Array int 32"=w1060:i32[][])  [unwired: 2 in, 2 out]
            n458 = Multiply(x=w1082, y=1.021) -> (x*y=w1096:dynamicdata)
            n459 = for {
              N -> [w1120]
              shift-right: [w1121] -> w1061
              shift-left: w1060 -> [w1122]
              tunnel: w1060 -> [w1115] mode=indexing
              i -> [w1116]
              n460 = Subtract(x=w1120, y=1) -> (x-y=w1118:i32)
              n461 = Subtract(x=w1118, y=w1116) -> (x-y=w1117:i32)
              n462 = Replace Array Subset(array=w1122, new element=w1115, index (row)=w1117) -> (w1121:i32[][])  [unwired: 1 in]
            }
            n463 = Greater?(x=w1094, y=u16 0) -> (0:w1080:bool)
            n464 = And(x=w1080, y=w1092) -> (x .and. y?=w1093:bool)
            n465 = call "WaitForBuffer.vi"("ph"=w1074, "sBufNr"=w1065, "sBufNr 2"=w1066, "timeout"=100, "error in (no error)"=w1073) -> ("hout"=w1076:u64, "error out"=w1103:errorcluster)  [unwired: 10 in, 3 out]
            n466 = Add(x=-0.5356, y=w1096) -> ()  [unwired: 1 out]
            n467 = call "GetImageBuffer2D.vi"("ph"=w1076, "BuffIn"=w1069, "BuffNr"=i16 0, "xRes"=w1068, "yRes"=w1067, "Bitresolution"=w1062) -> ("BuffOut"=w1056:u16[][])  [unwired: 6 in, 3 out]
            n468 = for {
              N -> [w1112]
              shift-right: [w1113] -> w1058
              shift-left: w1056 -> [w1114]
              tunnel: w1056 -> [w1107] mode=indexing
              i -> [w1108]
              n469 = Subtract(x=w1112, y=1) -> (x-y=w1110:i32)
              n470 = Subtract(x=w1110, y=w1108) -> (x-y=w1109:i32)
              n471 = Replace Array Subset(array=w1114, new element=w1107, index (row)=w1109) -> (w1113:u16[][])  [unwired: 1 in]
            }
            n472 = Transpose 2D Array(2D array=w1058) -> (transposed array=→"PixelFly Free Run":u16[][])
            n473 = Transpose 2D Array(2D array=w1061) -> (transposed array=→"CoolSnap Free Run":i32[][])
          }
        }
        frame 3 {
          (unwired) cluster{"date/time string":string, i32}[] []
          n474 = Unbundle(w1134) -> ("Camera Handle"=w1133:u32, "File Handle"=w1137:u32, "Display Handle"=w1136:u32, "Image Handle"=w1135:u32)
          n475 = while {
            tunnel: "error in (no error) 4" -> [w1173]
            tunnel: w1133 -> [w1172]
            tunnel: [w1170] -> _
            tunnel: w1137 -> [_]
            tunnel: w1136 -> [w1169]
            tunnel: w1135 -> [w1168]
            tunnel: [w1151] -> _
            tunnel: w1132 -> [w1165]
            tunnel: w1131 -> [w1162]
            tunnel: w1130 -> [w1161]
            tunnel: w1129 -> [w1160]
            tunnel: w1128 -> [w1158]
            tunnel: w1127 -> [w1159]
            tunnel: w1126 -> [w1154]
            tunnel: w1125 -> [w1157]
            tunnel: w1124 -> [w1156]
            tunnel: [w1154] -> w1123
            stop <- w1164 continue-if-true
            (unwired) 1
            # "Stop Button"
            # "ADC Inputs"
            n476 = Bundle(w1162, "XResAct"=w1161, "YResAct"=w1160, "BufNrOut"=w1159, "BufNrOut"=w1158, "ErrorOut"=w1157, "hout"=w1154, "Bits/pixel"=w1156) -> (w1155:T10)  [unwired: 1 in]
            n477 = call <userlib>:"CameraCheckData.vi"("Camera Handle"=w1172, "error in"=w1173) -> ("Camera Handle"=w1171:u32, "Number Of Frames Available"=w1167:i32)  [unwired: 1 out]
            n478 = control-ref of="?"() -> (w1150:refnum<vi>)
            n479 = Greater Or Equal?(x=w1167, y=1) -> (x >= y?=w1148:bool)
            n480 = property class="Bool (strict)"(reference=w1150) -> (error out=w1146:errorcluster, "Value"=w1149:bool)  [unwired: 1 in, 1 out]
            n481 = call "DAQ Assistant3"() -> ("data"=w1142:dynamicdata)  [unwired: 17 in, 2 out]
            n482 = case shown="True" w1148 {
              tunnel: w1171 -> [_ w1202]
              tunnel: [w1174 w1201] -> w1170
              tunnel: w1169 -> [_ w1200]
              tunnel: w1168 -> [_ w1199]
              tunnel: w1155 -> [_ w1198]
              tunnel: w1146 -> [w1174 _]
              frame False {
              }
              frame True {
                w1191 = 0
                (unwired) 1
                # "One shot only, bulb-triggered!"
                n483 = call <userlib>:"CameraGetData.vi"("Data Handle"=w1199, "Camera Handle"=w1202) -> ("error out"=w1197:errorcluster, "Data Handle"=w1196:u32)  [unwired: 1 in, 1 out]
                n484 = Unbundle(w1198) -> (w1188:u16[][], "XResAct"=w1187:u16, "YResAct"=w1186:u16, "BufNrOut"=w1185:i16, "BufNrOut"=w1184:i16, "ErrorOut"=w1183:errorcluster, "hout"=w1182:u64, "Bits/pixel"=w1181:u16)
                n485 = call <userlib>:"DisplayImage.vi"("error in"=w1197, "Image Handle"=w1196, "Display Handle"=w1200) -> ()  [unwired: 1 in, 2 out]
                n486 = call <userlib>:"ImageGetArrayI32.vi"("Image Handle"=w1196) -> ("Array int 32"=w1179:i32[][])  [unwired: 2 in, 2 out]
                n487 = for {
                  N -> [w1216]
                  shift-right: [w1217] -> w1180
                  shift-left: w1179 -> [w1218]
                  tunnel: w1179 -> [w1211] mode=indexing
                  i -> [w1212]
                  n488 = Subtract(x=w1216, y=1) -> (x-y=w1214:i32)
                  n489 = Subtract(x=w1214, y=w1212) -> (x-y=w1213:i32)
                  n490 = Replace Array Subset(array=w1218, new element=w1211, index (row)=w1213) -> (w1217:i32[][])  [unwired: 1 in]
                }
                n491 = call "AddBufferEX.vi"("ph"=w1182, "BuffNr"=i16 0, "1stImage"=w1191, "LastImage"=w1191, "error in (no error)"=w1183, "XRes"=w1187, "YRes"=w1186, "BitPerPixel"=w1181) -> ("hout"=w1193:u64, "error out"=w1192:errorcluster)  [unwired: 5 in, 1 out]
                n492 = call "WaitForBuffer.vi"("ph"=w1193, "sBufNr"=w1184, "sBufNr 2"=w1185, "timeout"=100, "error in (no error)"=w1192) -> ("hout"=w1195:u64, "error out"=w1201:errorcluster)  [unwired: 10 in, 3 out]
                n493 = call "GetImageBuffer2D.vi"("ph"=w1195, "BuffIn"=w1188, "BuffNr"=i16 0, "xRes"=w1187, "yRes"=w1186, "Bitresolution"=w1181) -> ("BuffOut"=w1177:u16[][])  [unwired: 6 in, 3 out]
                n494 = for {
                  N -> [w1208]
                  shift-right: [w1209] -> w1178
                  shift-left: w1177 -> [w1210]
                  tunnel: w1177 -> [w1203] mode=indexing
                  i -> [w1204]
                  n495 = Subtract(x=w1208, y=1) -> (x-y=w1206:i32)
                  n496 = Subtract(x=w1206, y=w1204) -> (x-y=w1205:i32)
                  n497 = Replace Array Subset(array=w1210, new element=w1203, index (row)=w1205) -> (w1209:u16[][])  [unwired: 1 in]
                }
                n498 = Transpose 2D Array(2D array=w1180) -> (transposed array=→"CoolSnap Single Shot":i32[][])
                n499 = Transpose 2D Array(2D array=w1178) -> (transposed array=→"PixelFly Single Shot":u16[][])
              }
            }
            n500 = Not(x=w1149) -> (.not. x?=w1163:bool)
            n501 = Greater?(x=w1165, y=u16 0) -> (0:w1152:bool)
            n502 = Multiply(x=w1142, y=1.021) -> (x*y=w1144:dynamicdata)
            n503 = And(x=w1152, y=w1163) -> (x .and. y?=w1164:bool)
            n504 = Add(x=-0.5356, y=w1144) -> (x+y=w1141:dynamicdata)
            n505 = local write "Top of Chamber Monitor"(w1141) -> ()
            n506 = Wait Until Next ms Multiple(millisecond multiple=1) -> (millisecond timer value=w1151:u32)
          }
        }
      }
      n507 = call "ExSubCloseExperimentCoolSnap.vi"("Handles In"=w69) -> ()  [unwired: 1 in, 1 out]
      n508 = call "CancelImages.vi"("ph"=w65) -> ("error out"=w68:errorcluster, "hout"=w67:u64)  [unwired: 2 in, 1 out]
      n509 = call "SetRecordingState.vi"("ErrorIn"=w68, "RecordingState"=w66, "ph"=w67) -> ("ErrorOut"=w60:errorcluster, "hout"=w61:u64)  [unwired: 2 in, 1 out]
      n510 = call "Cleanup.vi"("error in (no error)"=w60, "ph"=w61) -> ("error out"=w63:errorcluster, "hout"=w62:u64)  [unwired: 8 in]
      n511 = call "CloseCamera.vi"("ErrorIn"=w63, "Handle in"=w62) -> ("ErrorOut"=w64:errorcluster)  [unwired: 1 in, 2 out]
      n512 = call <vilib>:"Simple Error Handler.vi"("error in (no error)"=w64) -> ()  [unwired: 4 in, 5 out]
    }
  }
